vi "Photon Counter Control Panel big.vi"(8 "error in (no error)":errorcluster) -> (0 "error out":errorcluster)   [LabVIEW 2015]
uses:
  Public/Typedefs/Gate Mode.ctl
  Public/Typedefs/Discriminator Output.ctl
  <vilib>/Instr/_visa.llb/VISA GPIB Control REN Mode.ctl
  <vilib>/DAQmx/read.llb/DAQmx Read (Analog 1D DBL 1Chan NSamp).vi
  <vilib>/DAQmx/read.llb/DAQmx Read (Analog DBL 1Chan 1Samp).vi
  <vilib>/DAQmx/create/channels.llb/DAQmx Create Channel (AI-Voltage-Basic).vi
  <vilib>/Waveform/WDTFileIO.llb/Export Waveforms To Spreadsheet File (1D).vi
  <vilib>/DAQmx/miscellaneous.llb/DAQmx Fill In Error Info.vi
  SR400.lvlib
panel:
  out "PMT":dbl(graph)=0.0005292442580582076
  out "Wavemeter":dbl(graph)
  in  "file path":path=path "C:/Users/physics/Desktop/tessttt.xls"
  out "Scanning":bool
  out "Scan Finished":bool=TRUE
  out "Current Period":dbl=1.0
  out "Counter A":dbl(graph)=191.0
  out "Counter B":dbl(graph)
  in  "Monitor":bool
  in  "Start Scan":bool caption="Start Monitored Scan"
  in  "Stop Scan":bool
  out "Scan Start Time":timestamp=timestamp(3614449169.8747206 s since 1904-01-01)
  out "Counter A":dbl(graph)=5052.0
  out "Counter B":dbl(graph)=5104.0
  in  "Read Buffer Data":bool
  in  "Query Status Byte":bool
  out "Scan Start Time":timestamp=timestamp(3611333596.390047 s since 1904-01-01)
  in  "GPIB Address":i32=23 min=0 max=30 step=1
  in  "Stop Unmonitored Scan":bool
  in  "Disc A Mode":T1
  in  "Disc B Mode":T1
  in  "Disc B Slope":enum16{"Rise", "Fall"}(ring)
  in  "Disc A Slope":enum16{"Rise", "Fall"}(ring)
  in  "Trigger Slope":enum16{"Rise", "Fall"}(ring)
  in  "Set Gate Widths":bool
  in  "Set Gate Mode":bool
  out "Current":dbl[unit]=0.5 caption="Current Dwell Time"
  in  "Setpoint":dbl[unit]=0.5 caption="Dwell Time Target" min=0.0 max=60.0 step=0.5 format="%#_1g"
  in  "Set Dwell Time":bool
  in  "Setpoint":i32=5 caption="Number of Periods Target" min=0 max=2000 step=1
  out "Current":dbl=5.0 caption="Number of Periods Current"
  in  "Set # Periods":bool
  in  "Scan End Mode":enum16{"Stop", "Start"}(ring)
  in  "Disc B Lvl":dbl=-0.012 format="%#_13g"
  in  "Disc A Lvl":dbl=-0.012 format="%#_13g"
  in  "Display Mode":enum16{"Continuous", "Hold"}(ring)
  in  "Initialize":bool
  in  "Internal / External":bool
  in  "Set Count Time":bool
  in  "Counter B Input":enum16{"10 MHz", "INPUT 1", "INPUT 2", "TRIG"}(ring)=enum."INPUT 1"
  in  "Counter A Input":enum16{"10 MHz", "INPUT 1", "INPUT 2", "TRIG"}(ring)=enum."INPUT 1"
  in  "Count Mode":T2(ring)
  in  "Trigger Level":dbl=1.25 format="%#_13g"
  in  "VISA Resource Name":refnum<visa-resource-name>="GPIB0::23::INSTR"
  in  "Photon Counter SR 400":T3={"Mode"=0, "Count Time"=5.0, "Trigger Frequency"=10000000.0, "Trigger External?"=FALSE, "Gate A Mode"=0, "Gate A Width"=0.0002, "Gate A Delay"=0.0, "Gate B Mode"=0, "Gate B Width"=5e-09, "Gate B Delay"=0.0} {"Mode" items=["A,B For T Preset", "A-B For T Preset", "A+B For T Preset", "A For B Preset"]; "Gate A Mode" items=["CW", "Fixed"]; "Gate B Mode" items=["CW", "Fixed"]}
  out "Update visible/hidden":bool
  out "Current":T4
  out "Current":T4
  in  "stop":bool
  in  "Read to\nControl":bool
  in  "Read":bool
  out "Actual":dbl=200000.00000000003
  out "Actual":dbl=5.0
  in  "Target":dbl=5.0 caption="Gate A Width Percent Target"
  in  "Target":dbl=200000.00000000003 caption="Gate A Percent Target"
  in  "Gate Width: Time / Percent":bool caption="Time/Percent"
  in  "Start / Middle":bool
  in  "Setpoint":T4 caption="Gate B Mode Target"
  in  "Setpoint":T4 caption="Gate A Mode Target"
  out "Current":dbl[unit]=10000000.0 caption="Trigger Freq"
  in  "Setpoint":dbl[unit]=10000000.0 caption="Trigger Freq. Target"
  in  "Set Time & Freq.":bool
  in  "# Triggers vs Freq/Time":bool
  out "Current":dbl=50000000.0 caption="External Trigger # Cycles Current" format="%^#_6g"
  in  "Setpoint":dbl=50000000.0 format="%^#_6g"
  in  "Set # of Triggers":bool
  in  "Setpoint":dbl[unit]=5e-09 caption="Gate B Width Target"
  in  "Setpoint":dbl[unit]=0.0002 caption="Gate A Width Target"
  out "Current":dbl[unit]=0.0002 format="%^#_6g"
  out "Current":dbl[unit]=5e-09 format="%^#_6g"
  out "Current":dbl[unit]
  out "Current":dbl[unit]
  in  "Setpoint":dbl[unit]
  in  "Setpoint":dbl[unit] caption="Gate A Delay Target"
  in  "Set Gate Delays":bool
  in  "Start Unmonitored Scan":bool
  in  "Setpoint":dbl[unit]=5.0 caption="Count Time Target" min=0.0 step=0.5 format="%#_1f"
  out "Current":dbl[unit]=5.0 caption="Count Time Current" min=0.0 max=10000.0 step=1.0 format="%#_7g"
  # "SR400 Control Panel"
  # "Setup"
  # "Gates"
  # "Acquisition"
  # "Gate B Mode"
  # "# of Periods"
  # "Count Time"
  # "Gate A Mode"
  # "Gate A Width"
  # "Gate B Width"
  # "Dwell Time"
  # "Gate A Delay"
  # "Gate B Delay"
  # "Discriminator/Trigger"
  # "Set values and initialize.\n\nSettings you can \"live\" update w/o initialization:\n        All Gate Params\n        Count Time (Only largest sig digit used)\n        Dwell Time (Only largest sig digit used)\n        External Trigger\n        # Periods\n\nSettings without a \"Set _____\" button need to be changed by initialization.\n\nAll variables are initialized, but \"live\" params do not show current value until you press the set button for that parameter.\n\n\"Read\" sets the \"Current\" indicators to what the hardware has set.\n\n\"Read to Control\" sets the \"Setpoint\" controls to the values from \"Read\""
  # "Warning, saving data clears chart histories"
  # "External Trigger # of Cycles/Freq"
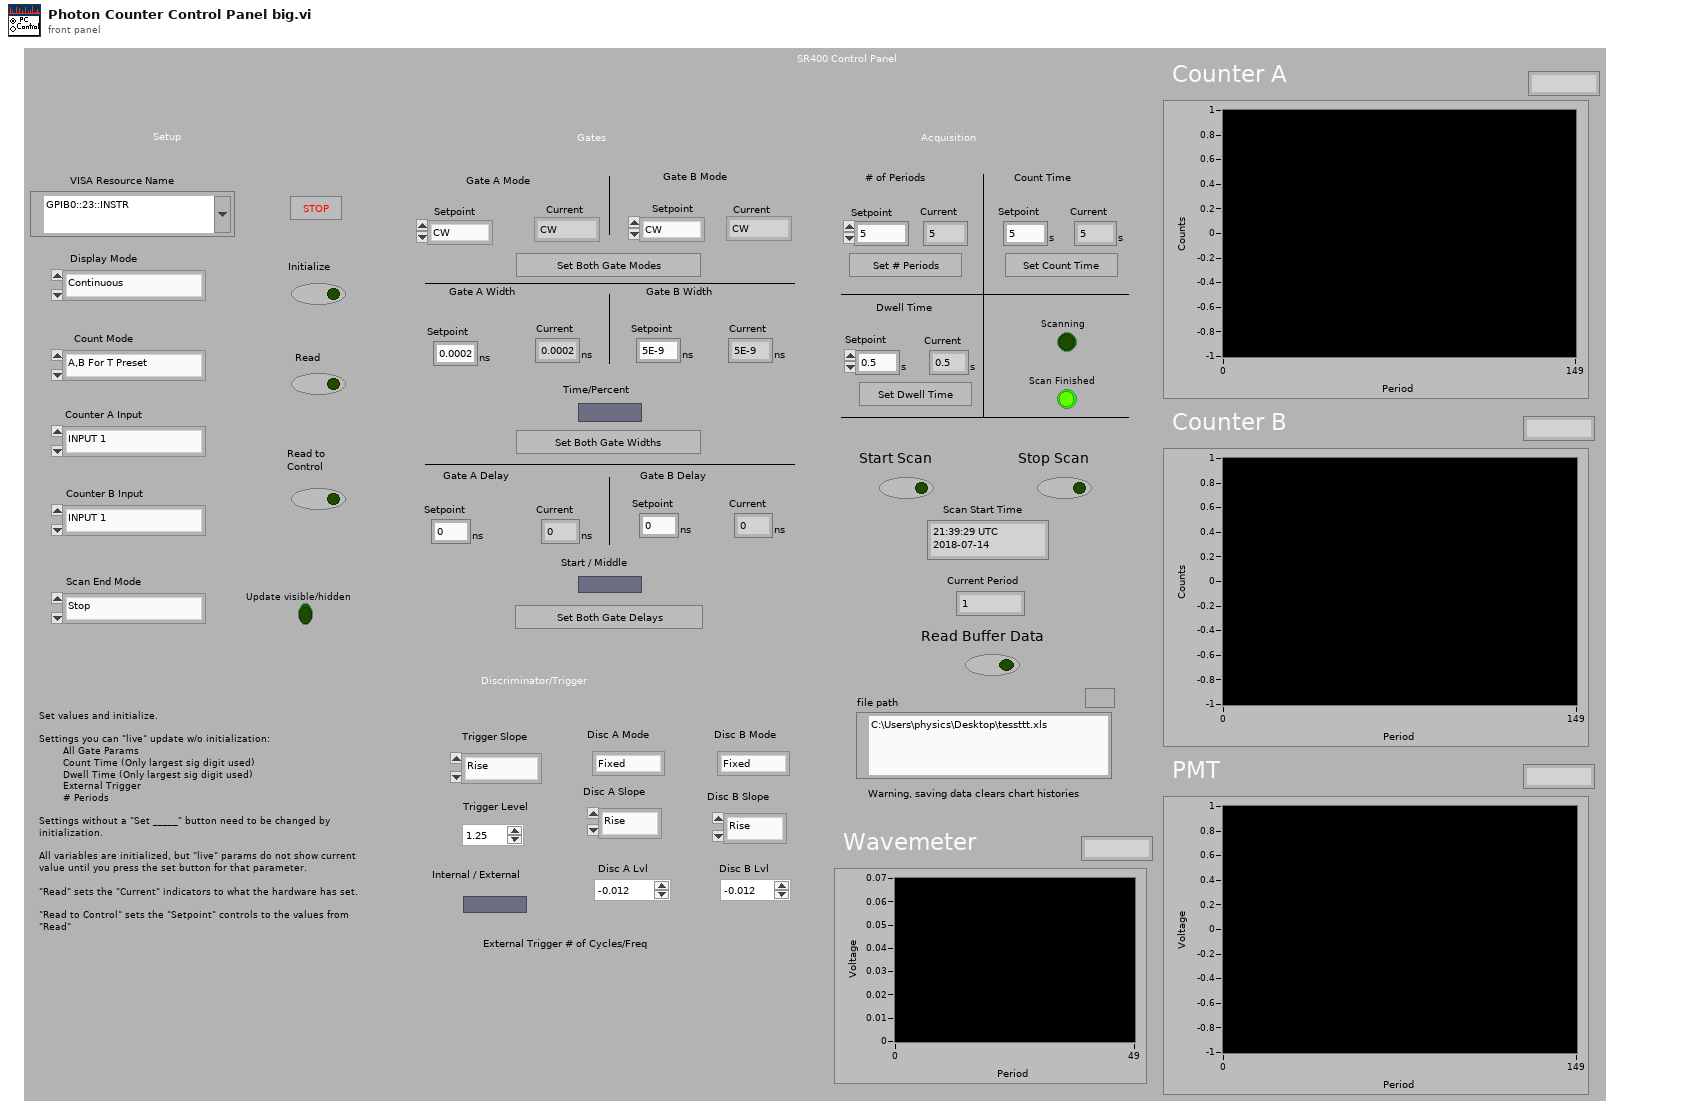
[diagram p1: front panel]
types:
  T1 = typedef "SR400.lvlib/Discriminator Output.ctl" = enum16{"Fixed", "Scan"}
  T2 = enum16{"A,B For T Preset", "A-B For T Preset", "A+B For T Preset", "A For B Preset"}
  T3 = cluster{"Mode":u16, "Count Time":dbl[unit], "Trigger Frequency":dbl[unit], "Trigger External?":bool, "Gate A Mode":u16, "Gate A Width":dbl[unit], "Gate A Delay":dbl[unit], "Gate B Mode":u16, "Gate B Width":dbl[unit], "Gate B Delay":dbl[unit]}
  T4 = typedef "SR400.lvlib/Gate Mode.ctl" = enum16{"CW", "Fixed", "Scan"}
  T5 = typedef "VISA GPIB Control REN Mode.ctl" = u16
  T6 = cluster{"Parameter Changed from front panel":bool, "Data Ready":bool, "Scan Finished":bool, "Counter Overrun":bool, "Rate Error":bool, "Recall Error":bool, "Service Request":bool, "Command Error":bool, "Triggered":bool, "Inhibited":bool, "Counting":bool}
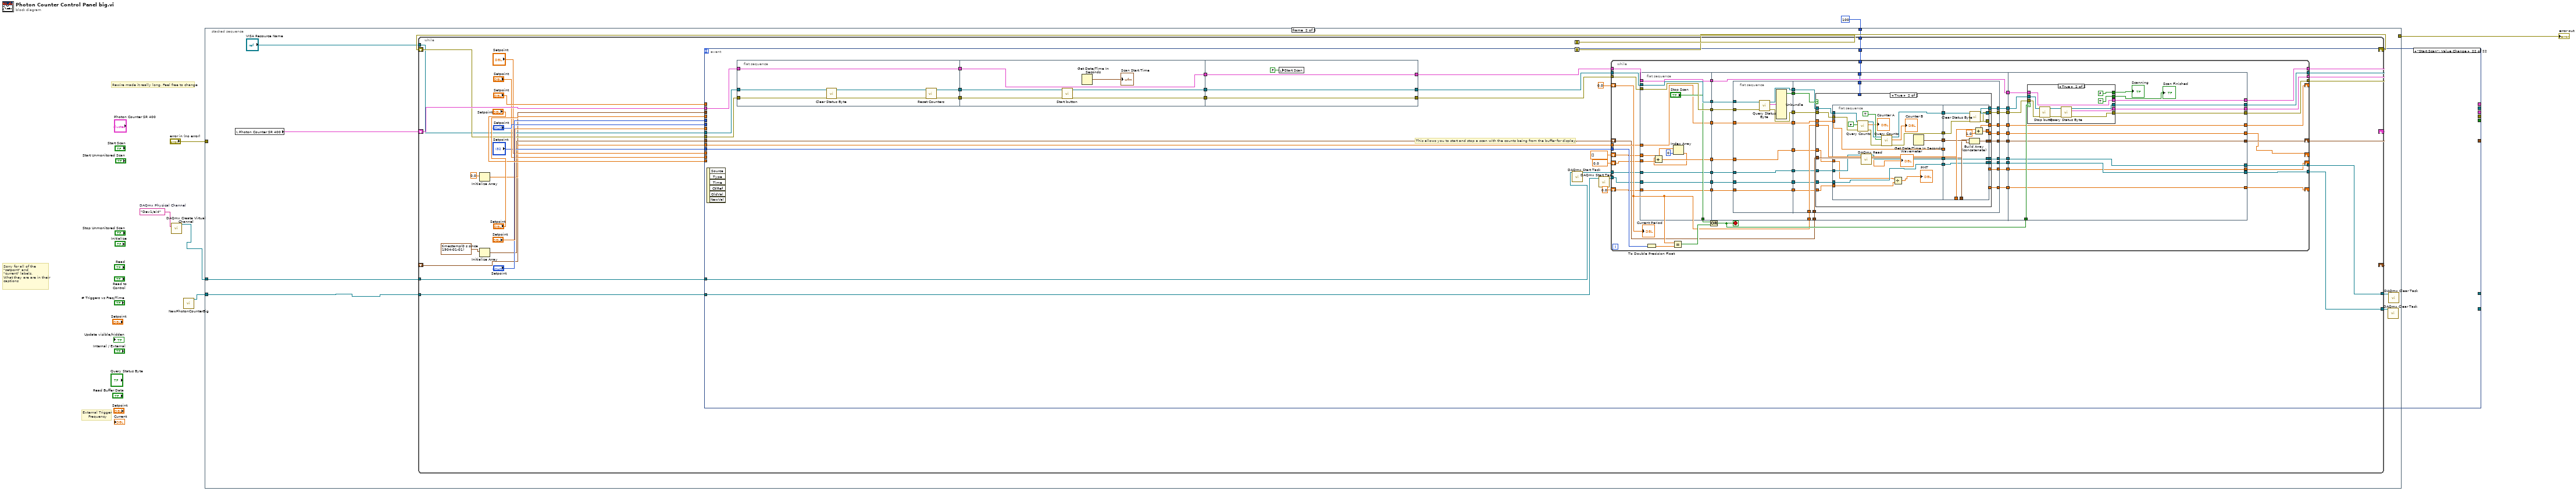
[diagram p0: block diagram]
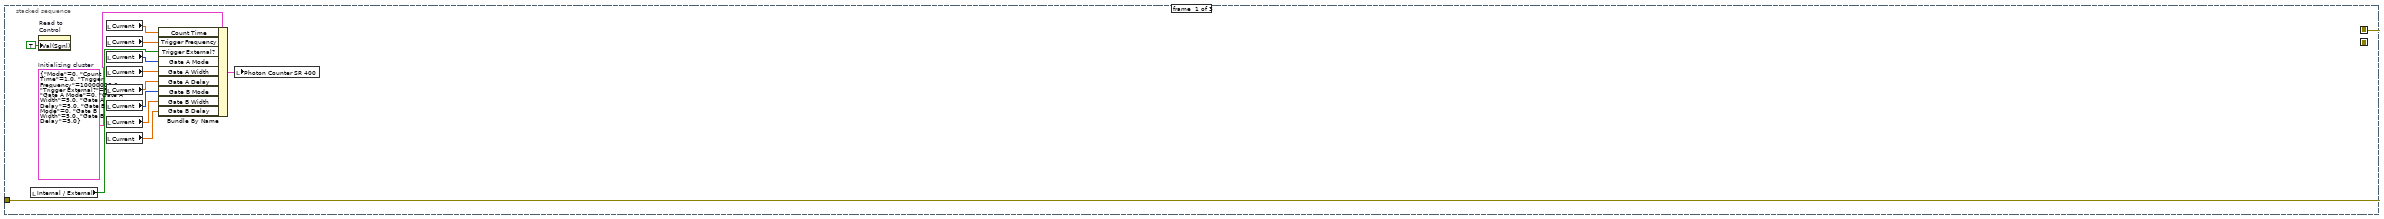
[diagram p2: hidden frame]
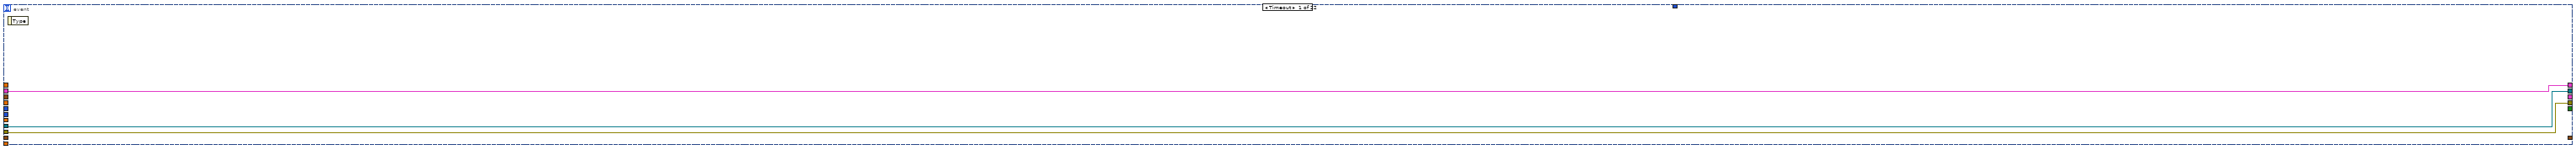
[diagram p3: hidden frame]
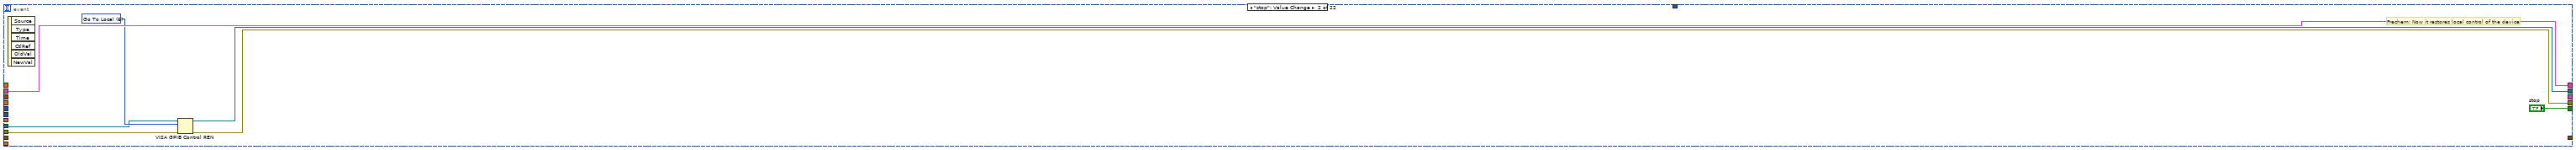
[diagram p4: hidden frame]
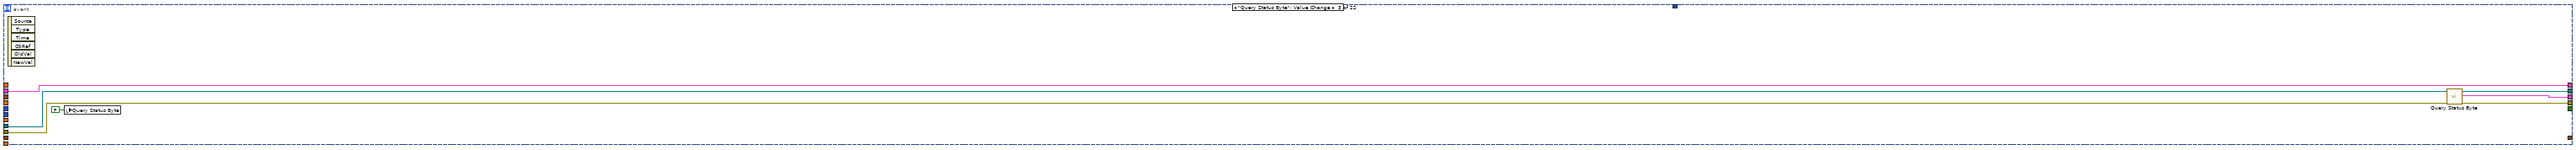
[diagram p5: hidden frame]
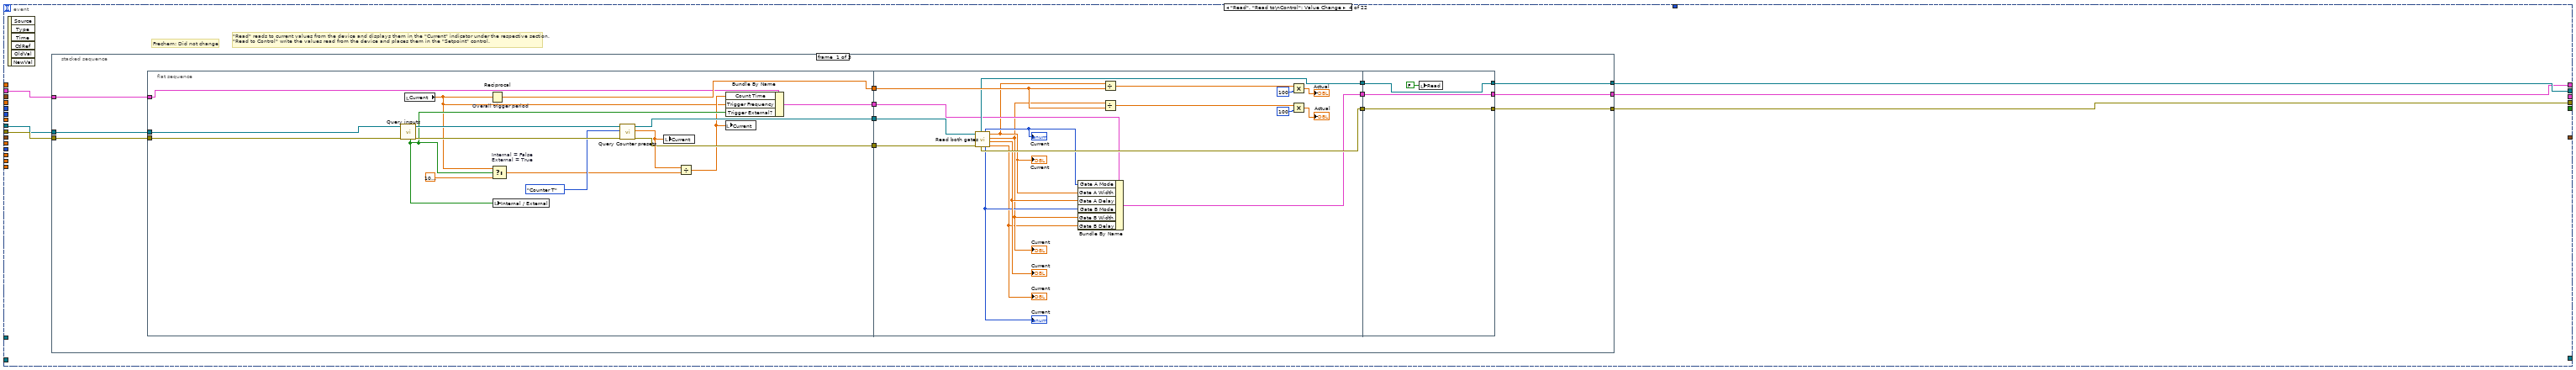
[diagram p6: hidden frame]
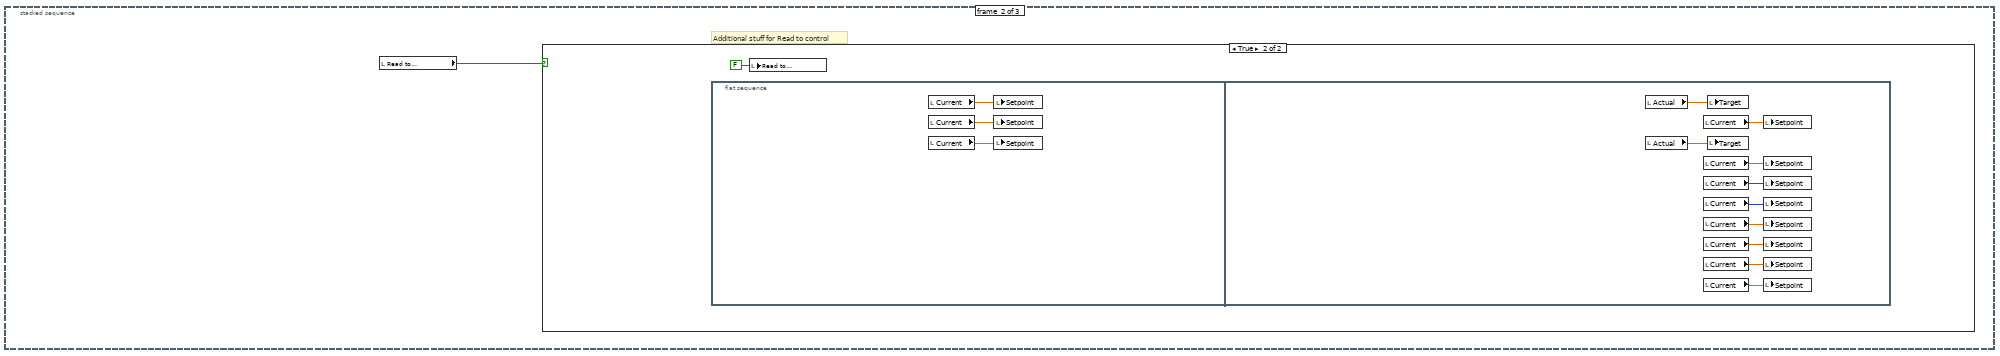
[diagram p7: hidden frame]
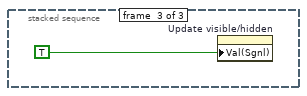
[diagram p9: hidden frame]
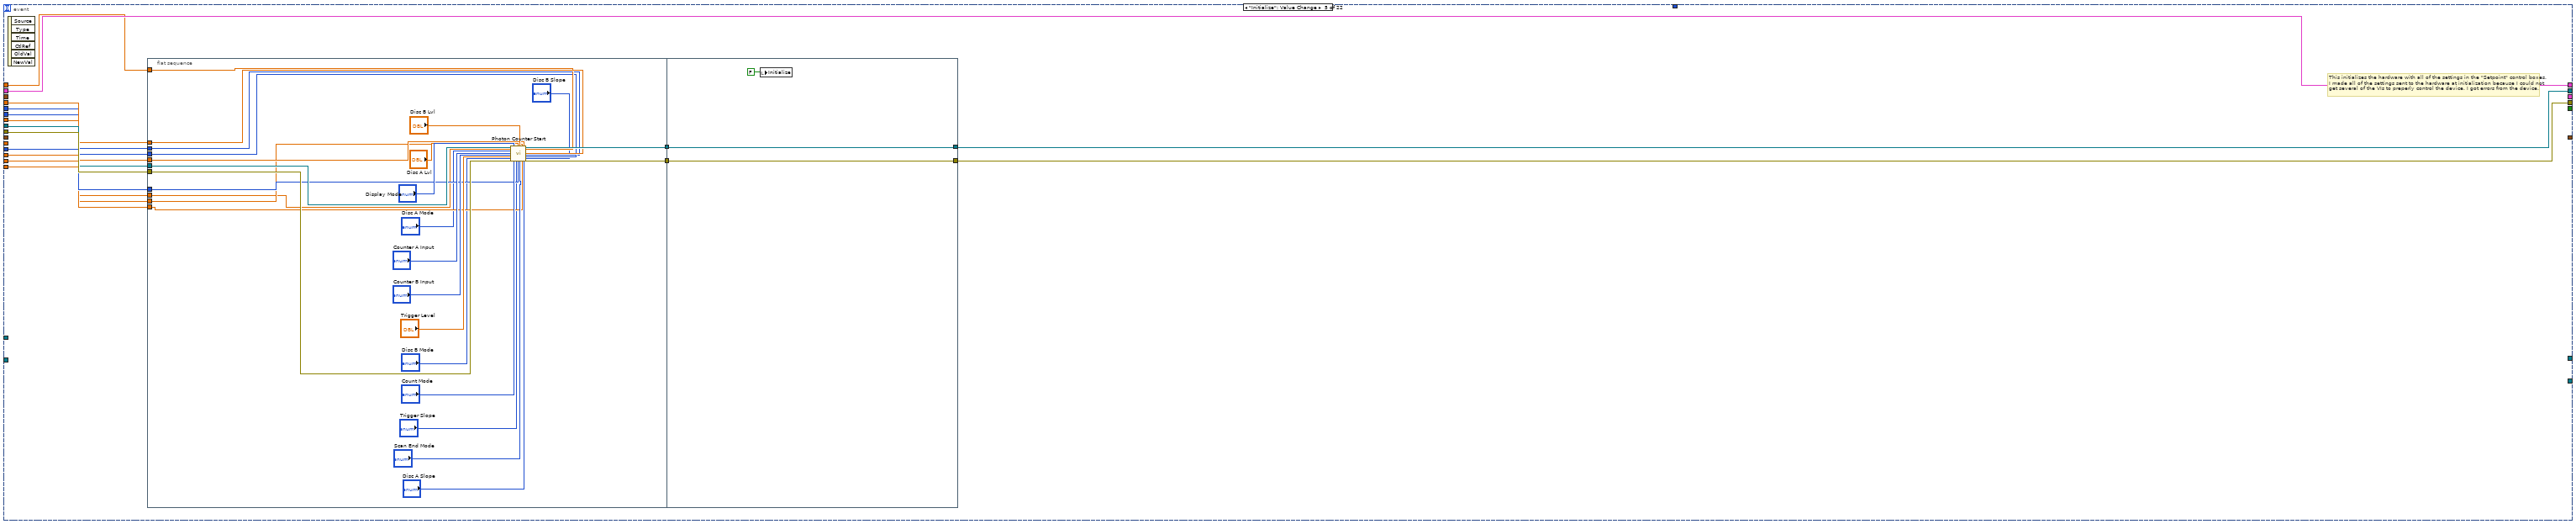
[diagram p10: hidden frame]
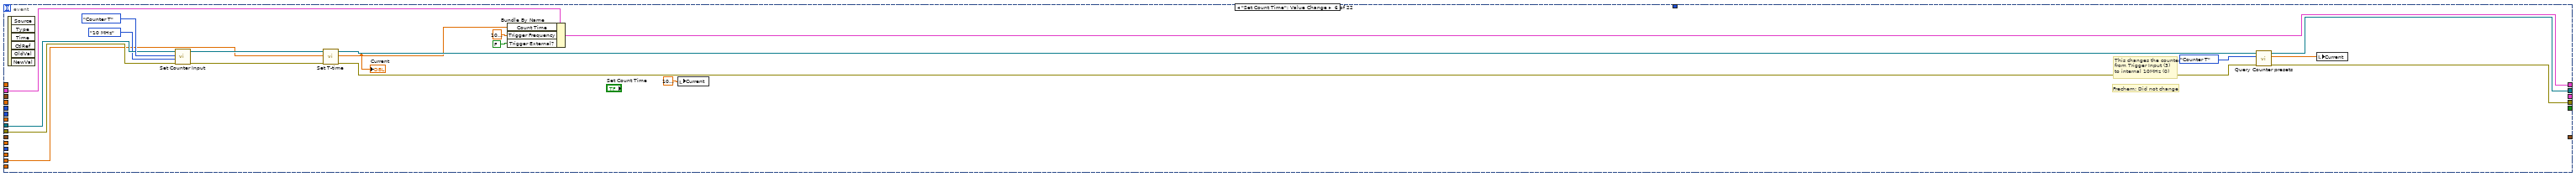
[diagram p11: hidden frame]
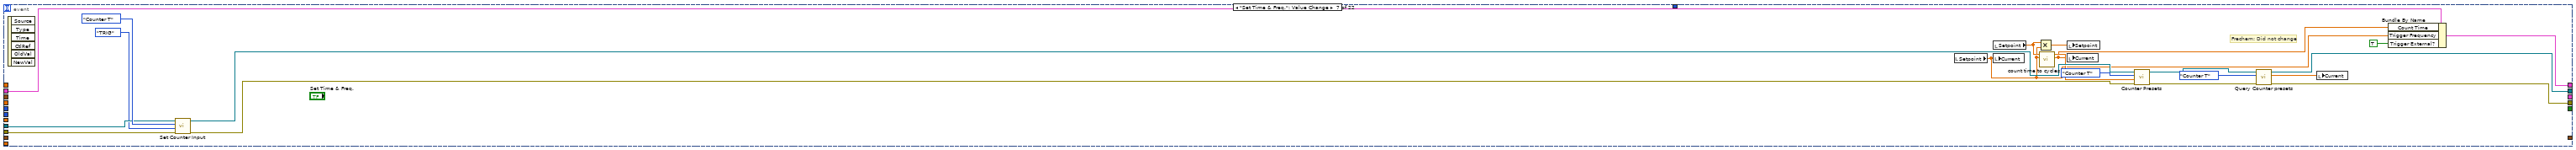
[diagram p12: hidden frame]
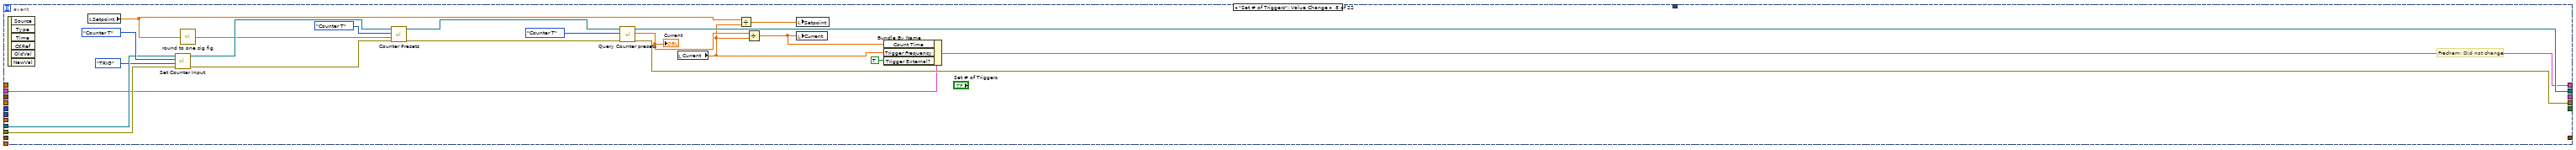
[diagram p13: hidden frame]
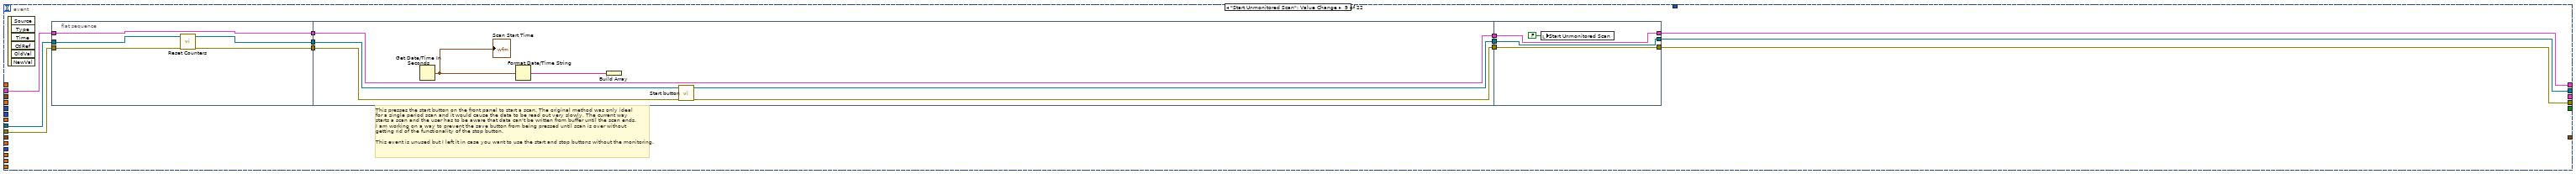
[diagram p14: hidden frame]
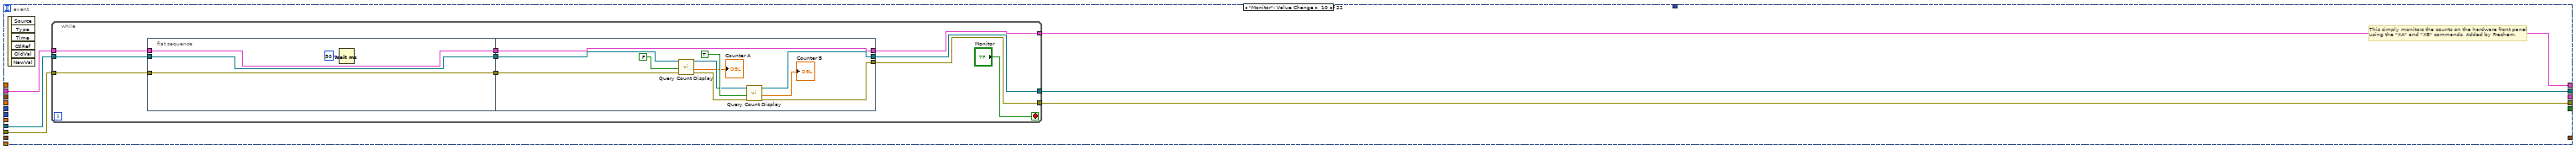
[diagram p15: hidden frame]
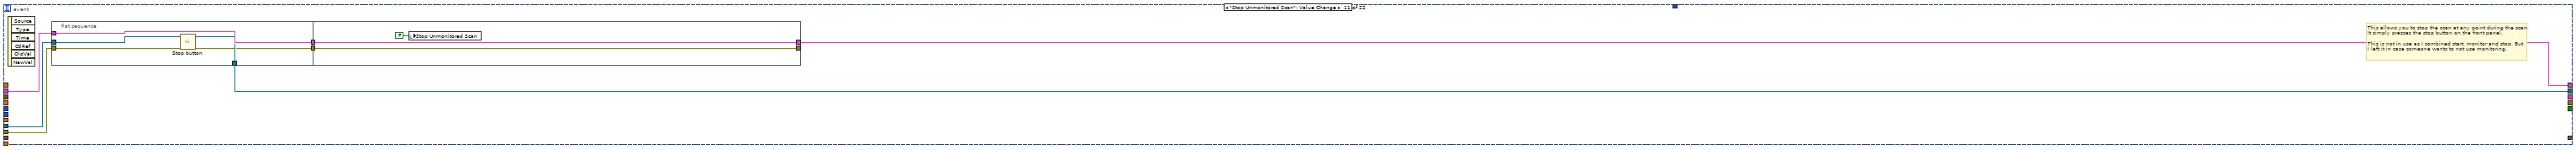
[diagram p16: hidden frame]
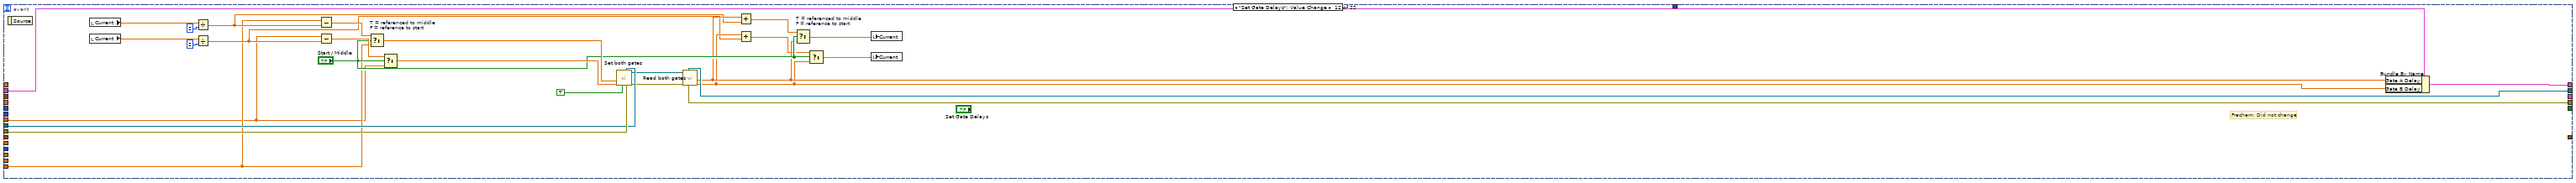
[diagram p17: hidden frame]
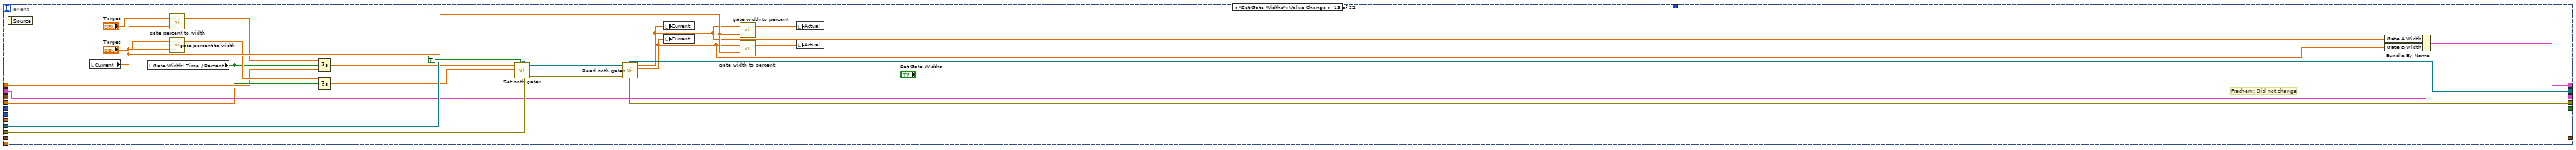
[diagram p18: hidden frame]
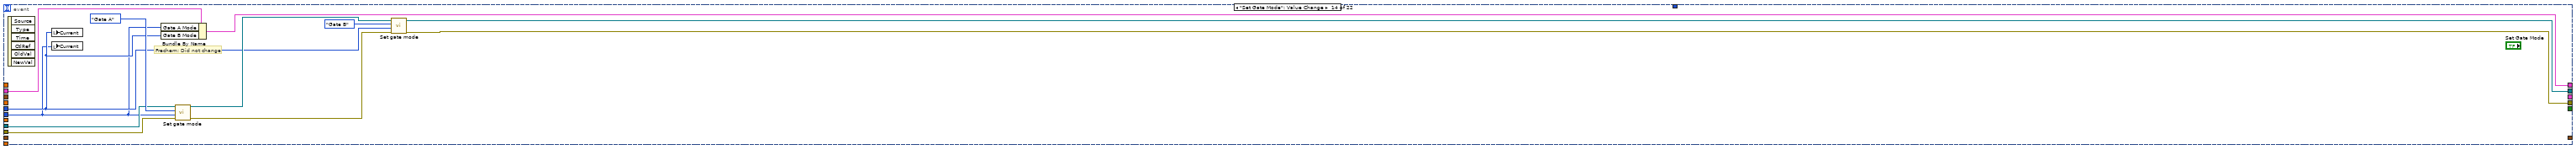
[diagram p19: hidden frame]
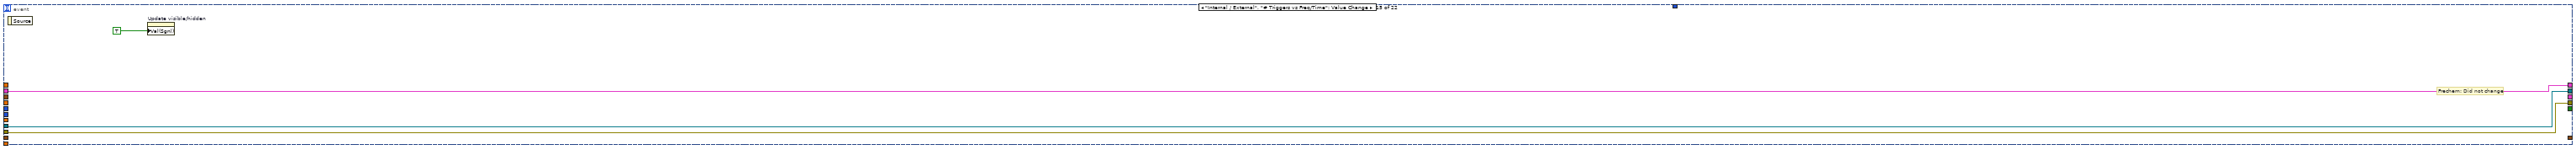
[diagram p20: hidden frame]
diagram:
  w2 = tag "Dev1/ai4"  # DAQmx Physical Channel
  # "Rewire made it really long. Feel free to change"
  # "Sorry for all of the\n\"setpont\" and \n\"current\" labels. \nWhat they are are in their\ncaptions"
  # "External Trigger \n     Frequency"
  n1 = call-poly <vilib>:"DAQmx Create Virtual Channel.vi"("physical channels"=w2) -> ("task out"=w1:refnum<k21>)  [unwired: 13 in, 1 out]
  n2 = call "NewPhotonCounterBig.vi"() -> ("task out"=w3:refnum<k21>)  [unwired: 10 in, 1 out]
  n3 = stacked-sequence {
    seq-local: [w9 _ _] -> [_ w28 _]
    seq-local: [_ w27 _] -> [_ _ w833]
    tunnel: "error in (no error)" -> [w9 _ _]
    tunnel: [_ _ w833] -> w5
    tunnel: 100 ("number of samples per channel") -> [_ w22 _]
    tunnel: w3 -> [_ w21 _]
    tunnel: w1 -> [_ w20 _]
    frame #0 {
      w7 = T3 {"Mode"=0, "Count Time"=1.0, "Trigger Frequency"=10000000.0, "Trigger External?"=FALSE, "Gate A Mode"=0, "Gate A Width"=5.0, "Gate A Delay"=5.0, "Gate B Mode"=0, "Gate B Width"=5.0, "Gate B Delay"=5.0}  # Initializing cluster
      n4 = local read "Internal / External"() -> (w16:bool)
      n5 = property on="Read to\nControl" class="Bool (strict)"("Val(Sgnl)"=TRUE ("Value (Signaling)")) -> ()  [unwired: 2 in, 2 out]
      n6 = local read "Current"() -> (w18:dbl[unit])
      n7 = local read "Current"() -> (w17:dbl[unit])
      n8 = local read "Current"() -> (w15:T4)
      n9 = local read "Current"() -> (w14:dbl[unit])
      n10 = local read "Current"() -> (w13:dbl[unit])
      n11 = local read "Current"() -> (w10:T4)
      n12 = local read "Current"() -> (w11:dbl[unit])
      n13 = local read "Current"() -> (w12:dbl[unit])
      n14 = Bundle By Name(cluster=w7, "Count Time"=w18, "Trigger Frequency"=w17, "Trigger External?"=w16, "Gate A Mode"=w15, "Gate A Width"=w14, "Gate A Delay"=w13, "Gate B Mode"=w10, "Gate B Width"=w11, "Gate B Delay"=w12) -> (w8:T3)
      n15 = local write "Photon Counter SR 400"(w8) -> ()
    }
    frame #1 {
      n16 = local read "Photon Counter SR 400"() -> (w26:T3)
      n17 = while {
        shift-right: [w52] -> _
        shift-left: w26 -> [w51]
        shift-right: [w54] -> w27
        shift-left: w28 -> [w42]
        tunnel: "VISA Resource Name" -> [w41]
        shift-right: [w35] -> _
        shift-left: _ -> [w34]
        tunnel: w20 -> [w33]
        tunnel: [w32] -> w24
        tunnel: [w31] -> w23
        tunnel: w21 -> [w30]
        tunnel: w22 -> [w29]
        stop <- w53 stop-if-true
        n18 = Initialize Array(0.0 ("element")) -> (w38:dbl[])  [unwired: 1 in]
        n19 = Initialize Array(timestamp(0 s since 1904-01-01)) -> (w36:timestamp[])  [unwired: 1 in]
        n20 = event shown="[21] \"Start Scan\": Value Change" {
          selector: _ -> [_ _ _ _ _ _ _ _ _ _ _ _ _ _ _ _ _ _ _ _ _ _]
          dyn-events: _ -> [_ _ _ _ _ _ _ _ _ _ _ _ _ _ _ _ _ _ _ _ _ _]
          timeout: _ -> [_ _ _ _ _ _ _ _ _ _ _ _ _ _ _ _ _ _ _ _ _ _]
          tunnel: [w57 w59 w67 w76 w158 w208 w226 w250 w260 w285 w313 w340 w372 w382 w393 w396 w422 w455 w471 w478 w503 w582] -> _
          tunnel: w42 -> [w56 w62 w69 w78 w162 w199 w220 w242 w264 w284 w316 w354 w373 w386 w392 w394 w421 w454 w468 w484 w506 w585]
          tunnel: [w56 w61 w68 w75 w161 w207 w227 w249 w262 w286 _ w338 w371 w383 w392 w395 w421 w454 w470 w477 w505 w584] -> w55
          tunnel: w41 -> [w57 w60 w70 w77 w156 w200 w221 w243 w256 w283 w315 w353 w374 w387 w393 w396 w422 w455 w469 w485 w504 w586]
          tunnel: w51 -> [w58 w64 w72 w74 w157 w197 w215 w236 w258 w282 w314 w352 w360 w381 w391 w397 w423 w453 w467 w476 w502 w587]
          tunnel: [w58 w64 w72 w73 w157 w196 w214 w235 w257 w281 w312 w351 w359 w380 w391 w397 w423 w453 w467 w476 w501 w583] -> w52
          tunnel: [_ "stop" _ _ _ _ _ _ _ _ _ _ _ _ _ _ _ _ _ _ _ _] -> w53
          tunnel: "Setpoint" -> [_ _ _ _ w155 _ _ _ _ _ _ _ _ _ _ _ _ _ w466 _ w500 w578]
          tunnel: "Setpoint" -> [_ _ _ _ w154 _ _ _ _ _ _ _ w356 _ _ _ _ _ _ _ _ _]
          tunnel: "Setpoint" -> [_ _ _ _ w153 _ _ _ _ _ _ _ w355 _ _ _ _ _ _ _ _ _]
          tunnel: "Setpoint" -> [_ _ _ _ w152 _ _ _ _ _ _ w328 _ _ _ _ _ _ _ _ _ _]
          tunnel: "Setpoint" -> [_ _ _ _ w151 _ _ _ _ _ _ w327 _ _ _ _ _ _ _ _ _ _]
          tunnel: "Setpoint" -> [_ _ _ _ w150 w192 _ _ _ _ _ _ _ _ _ _ _ _ _ _ w488 _]
          tunnel: "Setpoint" -> [_ _ _ _ w148 _ _ _ _ _ _ _ _ w379 _ _ _ _ _ _ _ _]
          tunnel: "Setpoint" -> [_ _ _ _ w149 _ _ _ _ _ _ _ _ w378 _ _ _ _ _ _ _ _]
          tunnel: "Setpoint" -> [_ _ _ _ w147 _ _ _ _ _ _ _ _ _ _ _ _ _ _ w482 w489 _]
          tunnel: [_ _ w66 _ _ _ _ _ _ _ _ _ _ _ _ _ _ _ _ _ _ w581] -> _
          tunnel: w38 -> [_ _ _ _ _ _ _ _ _ _ _ _ _ _ _ _ _ _ _ _ _ w579]
          tunnel: w36 -> [_ _ _ _ _ _ _ _ _ _ _ _ _ _ _ _ _ _ _ _ _ w577]
          tunnel: [_ _ _ _ _ _ _ _ _ _ _ _ _ _ _ _ _ _ _ _ _ w576] -> w35
          tunnel: w34 -> [_ _ _ _ _ _ _ _ _ _ _ _ _ _ _ _ _ _ _ _ w490 _]
          tunnel: w33 -> [_ _ _ _ _ _ _ _ _ _ _ _ _ _ _ _ _ _ _ _ _ w567]
          tunnel: [_ _ _ _ _ _ _ _ _ _ _ _ _ _ _ _ _ _ _ _ _ w575] -> w32
          tunnel: [_ _ _ _ _ _ _ _ _ _ _ _ _ _ _ _ _ _ _ _ _ w574] -> w31
          tunnel: w30 -> [_ _ _ _ _ _ _ _ _ _ _ _ _ _ _ _ _ _ _ _ _ w569]
          tunnel: w29 -> [_ _ _ _ _ _ _ _ _ _ _ _ _ _ _ _ _ _ _ _ _ w573]
          event Timeout {
            n21 = event-data() -> ()  [unwired: 2 out]
          }
          event "stop": Value Change {
            w63 = T5 6 items=["Deassert REN", "Assert REN", "Go To Local; Deassert REN ", "Assert REN; Address Device", "Local Lockout (Addressed Devices)", "Local Lockout (This Device)", "Go To Local"] ("Mode")
            # "Frechem: Now it restores local control of the device"
            n22 = event-data() -> ()  [unwired: 7 out]
            n23 = VISA GPIB Control REN(8:w62, 10:w63, 11:w60) -> (0:w61:errorcluster, 3:w59:refnum<visa-resource-name>)
          }
          event "Query Status Byte": Value Change {
            n24 = event-data() -> ()  [unwired: 7 out]
            n25 = local write "Query Status Byte"(FALSE ("Read Channels")) -> ()
            n26 = call "Query Status Byte.vi"("error in (no error)"=w69, "VISA resource name"=w70) -> ("error out"=w68:errorcluster, "Status Register"=w66:T6, "VISA resource name out"=w67:refnum<visa-resource-name>)  [unwired: 7 in]
          }
          event "Read", "Read to\nControl": Value Change {
            # "Frechem: Did not change"
            # "\"Read\" reads to current values from the device and displays them in the \"Current\" indicator under the respective section.\n\"Read to Control\" write the values read from the device and places them in the \"Setpoint\" control."
            n27 = event-data() -> ()  [unwired: 7 out]
            n28 = stacked-sequence {
              tunnel: w78 -> [w90 _ _]
              tunnel: w77 -> [w91 _ _]
              tunnel: [w86 _ _] -> w76
              tunnel: [w84 _ _] -> w75
              tunnel: w74 -> [w82 _ _]
              tunnel: [w80 _ _] -> w73
              frame #0 {
                n29 = flat-sequence {
                  tunnel: w91 -> [w107]
                  tunnel: w90 -> [w104]
                  tunnel: [w100] -> w89
                  tunnel: [w99] -> w88
                  tunnel: [w98] -> w87
                  tunnel: w82 -> [w96]
                  tunnel: [w92] -> w81
                  tunnel: w89 -> [w120]
                  tunnel: w88 -> [w119]
                  tunnel: w87 -> [w118]
                  tunnel: [w117] -> w85
                  tunnel: [w116] -> w83
                  tunnel: w81 -> [w115]
                  tunnel: [w108] -> w79
                  tunnel: [w129] -> w86
                  tunnel: w85 -> [w129]
                  tunnel: [w128] -> w84
                  tunnel: w83 -> [w128]
                  tunnel: [w127] -> w80
                  tunnel: w79 -> [w127]
                  frame #0 {
                    n30 = call "Query inputs.vi"("error in (no error)"=w104, "VISA resource name"=w107) -> ("error out"=w105:errorcluster, "VISA resource name out"=w106:refnum<visa-resource-name>, "Externally-triggered?"=w95:bool)  [unwired: 7 out]
                    n31 = local read "Current"() -> (w93:dbl[unit])
                    n32 = Reciprocal "Overall trigger period"(x=w93) -> (1/x=w98:dbl[unit])
                    n33 = Select "Internal = False\nExternal = True"(t=w93, s=w95, f=dbl[unit] 10000000.0 ("freq")) -> (s? t:f=w102:dbl[unit])
                    n34 = local write "Internal / External"(w95) -> ()
                    n35 = call "Query Counter presets.vi"("error in (no error)"=w105, "Counter (Def: T)"=enum16{"Invalid", "Counter B", "Counter T"}."Counter T" ("i (0)"), "VISA resource name"=w106) -> ("error out"=w99:errorcluster, "Number of triggers"=w101:dbl, "VISA resource name out"=w100:refnum<visa-resource-name>)  [unwired: 6 out]
                    n36 = local write "Current"(w101) -> ()
                    n37 = Divide(x=w101, y=w102) -> (x/y=w94:dbl[unit])
                    n38 = Bundle By Name(cluster=w96, "Count Time"=w94, "Trigger Frequency"=w93, "Trigger External?"=w95) -> (w92:T3)
                    n39 = local write "Current"(w94) -> ()
                  }
                  frame #1 {
                    n40 = call "Read both gates.vi"("error in (no error)"=w119, "VISA resource name"=w120) -> ("Gate B Delay"=w109:dbl[unit], "Gate A Delay"=w112:dbl[unit], "Gate B Width"=w110:dbl[unit], "Gate A Width"=w113:dbl[unit], "Current mode B"=w111:enum16{"CW", "Fixed", "Scan"}, "Current mode A"=w114:enum16{"CW", "Fixed", "Scan"}, "error out"=w116:errorcluster, "VISA resource name out"=w117:refnum<visa-resource-name>)  [unwired: 2 out]
                    "Current" <- w110
                    "Current" <- w113
                    "Current" <- w112
                    "Current" <- w109
                    "Current" <- w114
                    "Current" <- w111
                    n41 = Bundle By Name(cluster=w115, "Gate A Mode"=w114, "Gate A Width"=w113, "Gate A Delay"=w112, "Gate B Mode"=w111, "Gate B Width"=w110, "Gate B Delay"=w109) -> (w108:T3)
                    n42 = Divide(x=w113, y=w118) -> (x/y=w122:dbl)
                    n43 = Divide(x=w110, y=w118) -> (x/y=w124:dbl)
                    n44 = Multiply(x=w122, y=i8 100) -> (x*y=→"Actual":dbl)
                    n45 = Multiply(x=w124, y=i8 100) -> (x*y=→"Actual":dbl)
                  }
                  frame #2 {
                    n46 = local write "Read"(FALSE ("Read")) -> ()
                  }
                }
              }
              frame #1 {
                # "Additional stuff for Read to control"
                n47 = local read "Read to\nControl"() -> (w131:bool)
                n48 = case shown="True" w131 {
                  frame False {
                  }
                  frame True {
                    n49 = flat-sequence {
                      frame #0 {
                        n50 = local read "Current"() -> (w134:dbl)
                        n51 = local read "Current"() -> (w133:dbl[unit])
                        n52 = local read "Current"() -> (w135:dbl[unit])
                        n53 = local write "Setpoint"(w134) -> ()
                        n54 = local write "Setpoint"(w133) -> ()
                        n55 = local write "Setpoint"(w135) -> ()
                      }
                      frame #1 {
                        n56 = local read "Actual"() -> (w142:dbl)
                        n57 = local read "Actual"() -> (w144:dbl)
                        n58 = local read "Current"() -> (w137:dbl[unit])
                        n59 = local read "Current"() -> (w138:dbl[unit])
                        n60 = local read "Current"() -> (w140:T4)
                        n61 = local read "Current"() -> (w139:T4)
                        n62 = local read "Current"() -> (w143:dbl[unit])
                        n63 = local read "Current"() -> (w141:dbl[unit])
                        n64 = local read "Current"() -> (w145:dbl[unit])
                        n65 = local read "Current"() -> (w136:dbl[unit])
                        n66 = local write "Target"(w142) -> ()
                        n67 = local write "Target"(w144) -> ()
                        n68 = local write "Setpoint"(w137) -> ()
                        n69 = local write "Setpoint"(w138) -> ()
                        n70 = local write "Setpoint"(w140) -> ()
                        n71 = local write "Setpoint"(w139) -> ()
                        n72 = local write "Setpoint"(w143) -> ()
                        n73 = local write "Setpoint"(w141) -> ()
                        n74 = local write "Setpoint"(w145) -> ()
                        n75 = local write "Setpoint"(w136) -> ()
                      }
                    }
                    n76 = local write "Read to\nControl"(FALSE ("Read to Control")) -> ()
                  }
                }
              }
              frame #2 {
                n77 = property on="Update visible/hidden" class="Bool (strict)"("Val(Sgnl)"=TRUE ("Value (Signaling)")) -> ()  [unwired: 2 in, 2 out]
              }
            }
          }
          event "Initialize": Value Change {
            # "This initializes the hardware with all of the settings in the \"Setpoint\" control boxes.\nI made all of the settings sent to the hardware at initialization because I could not \nget several of the VIs to preperly control the device. I got errors from the device."
            n78 = event-data() -> ()  [unwired: 7 out]
            n79 = flat-sequence {
              tunnel: w162 -> [w188]
              tunnel: [w187] -> w160
              tunnel: [w186] -> w159
              tunnel: w156 -> [w185]
              tunnel: w155 -> [w176]
              tunnel: w154 -> [w175]
              tunnel: w153 -> [w174]
              tunnel: w152 -> [w173]
              tunnel: w151 -> [w172]
              tunnel: w150 -> [w171]
              tunnel: w149 -> [w170]
              tunnel: w148 -> [w169]
              tunnel: w147 -> [w168]
              tunnel: [w190] -> w161
              tunnel: [w191] -> w158
              tunnel: w160 -> [w191]
              tunnel: w159 -> [w190]
              frame #0 {
                n80 = call "Photon Counter Start.vi"("VISA resource name"=w185, "Dwell Time"=w168, "Disc A Mode"="Disc A Mode", "Count A Input"="Counter A Input", "Count B Input"="Counter B Input", "Trigger Level"="Trigger Level", "Disc B Mode"="Disc B Mode", "errorIN"=w188, "Display Mode"="Display Mode", "Count Mode"="Count Mode", "Trigger Slope"="Trigger Slope", "Disc A Lvl"="Disc A Lvl", "# of periods"=w176, "Disc B Lvl"="Disc B Lvl", "Scan End Mode"="Scan End Mode", "Count Time Set"=w171, "Gate A Delay (def: 0 s)"=w173, "Gate B Delay (def: 0 s)"=w172, "Disc A\nSlope"="Disc A Slope", "Gate A Width (def: 0 s)"=w174, "Gate B Width (def: 0 s)"=w175, "Gate B Mode"=w169, "Gate A Mode"=w170, "Disc B\nSlope"="Disc B Slope") -> ("VISA resource name out"=w187:refnum<visa-resource-name>, "errorOUT"=w186:errorcluster)  [unwired: 2 in]
              }
              frame #1 {
                n81 = local write "Initialize"(FALSE ("Re-initialize")) -> ()
              }
            }
          }
          event "Set Count Time": Value Change {
            # "Frechem: Did not change"
            # "This changes the counters\nfrom Trigger Input (3)\nto internal 10MHz (0)"
            n82 = event-data() -> ()  [unwired: 7 out]
            n83 = call "Set Counter Input.vi"("error in (no error)"=w199, "Input (def: 10 MHz)"=enum16{"10 MHz", "INPUT 1", "INPUT 2", "TRIG"}."10 MHz" ("n (0.000000)"), "Counter (def: A)"=enum16{"Counter A", "Counter B", "Counter T"}."Counter T" ("i (0) 2"), "VISA resource name"=w200) -> ("error out"=w202:errorcluster, "VISA resource name out"=w201:refnum<visa-resource-name>)  [unwired: 6 out]
            n84 = call "Set T-time.vi"("errorIN"=w202, "Count Time Set"=w192, "VISA resource name"=w201) -> ("errorOUT"=w203:errorcluster, "ttimeOUT"=w195:dbl[unit], "VISA resource name out"=w206:refnum<visa-resource-name>)  [unwired: 4 out]
            "Current" <- w195
            n85 = Bundle By Name(cluster=w197, "Count Time"=w195, "Trigger Frequency"=dbl[unit] 10000000.0, "Trigger External?"=FALSE) -> (w196:T3)
            n86 = local write "Current"(dbl[unit] 10000000.0 ("freq")) -> ()
            n87 = call "Query Counter presets.vi"("error in (no error)"=w203, "Counter (Def: T)"=enum16{"Invalid", "Counter B", "Counter T"}."Counter T" ("i (0)"), "VISA resource name"=w206) -> ("error out"=w207:errorcluster, "Number of triggers"=w209:dbl, "VISA resource name out"=w208:refnum<visa-resource-name>)  [unwired: 6 out]
            n88 = local write "Current"(w209) -> ()
          }
          event "Set Time & Freq.": Value Change {
            # "Frechem: Did not change"
            n89 = event-data() -> ()  [unwired: 7 out]
            n90 = call "Set Counter Input.vi"("error in (no error)"=w220, "Input (def: 10 MHz)"=enum16{"10 MHz", "INPUT 1", "INPUT 2", "TRIG"}."TRIG" ("n (0.000000)"), "Counter (def: A)"=enum16{"Counter A", "Counter B", "Counter T"}."Counter T" ("i (0) 2"), "VISA resource name"=w221) -> ("error out"=w222:errorcluster, "VISA resource name out"=w223:refnum<visa-resource-name>)  [unwired: 6 out]
            n91 = local read "Setpoint"() -> (w211:dbl[unit])
            n92 = local read "Setpoint"() -> (w216:dbl[unit])
            n93 = local write "Current"(w211) -> ()
            n94 = Multiply(x=w216, y=w211) -> (x*y=w217:dbl)
            n95 = call "count time to cycles.vi"("Trigger Freq"=w211, "Count Time Set"=w216) -> ("Count Time Current"=w212:dbl[unit], "Number of triggers"=w218:dbl)  [unwired: 3 in, 1 out]
            n96 = local write "Setpoint"(w217) -> ()
            n97 = local write "Current"(w212) -> ()
            n98 = call "Counter Presets.vi"("error in (no error)"=w222, "Number of triggers"=w218, "Counter (Def: T)"=enum16{"Invalid", "Counter B", "Counter T"}."Counter T" ("i (0) 2"), "VISA resource name"=w223) -> ("error out"=w228:errorcluster, "VISA resource name out"=w225:refnum<visa-resource-name>)  [unwired: 6 out]
            n99 = call "Query Counter presets.vi"("error in (no error)"=w228, "Counter (Def: T)"=enum16{"Invalid", "Counter B", "Counter T"}."Counter T" ("i (0)"), "VISA resource name"=w225) -> ("error out"=w227:errorcluster, "Number of triggers"=w229:dbl, "VISA resource name out"=w226:refnum<visa-resource-name>)  [unwired: 6 out]
            n100 = local write "Current"(w229) -> ()
            n101 = Bundle By Name(cluster=w215, "Count Time"=w212, "Trigger Frequency"=w211, "Trigger External?"=TRUE) -> (w214:T3)
          }
          event "Set # of Triggers": Value Change {
            # "Frechem: Did not change"
            n102 = event-data() -> ()  [unwired: 7 out]
            n103 = local read "Setpoint"() -> (w240:dbl)
            n104 = call "Set Counter Input.vi"("error in (no error)"=w242, "Input (def: 10 MHz)"=enum16{"10 MHz", "INPUT 1", "INPUT 2", "TRIG"}."TRIG" ("n (0.000000)"), "Counter (def: A)"=enum16{"Counter A", "Counter B", "Counter T"}."Counter T" ("i (0) 2"), "VISA resource name"=w243) -> ("error out"=w244:errorcluster, "VISA resource name out"=w245:refnum<visa-resource-name>)  [unwired: 6 out]
            n105 = call "round to one sig fig.vi"("input number"=w240) -> ("rounded to 1 sig fig"=w238:dbl)
            n106 = call "Counter Presets.vi"("error in (no error)"=w244, "Number of triggers"=w238, "Counter (Def: T)"=enum16{"Invalid", "Counter B", "Counter T"}."Counter T" ("i (0) 2"), "VISA resource name"=w245) -> ("error out"=w248:errorcluster, "VISA resource name out"=w247:refnum<visa-resource-name>)  [unwired: 6 out]
            n107 = call "Query Counter presets.vi"("error in (no error)"=w248, "Counter (Def: T)"=enum16{"Invalid", "Counter B", "Counter T"}."Counter T" ("i (0)"), "VISA resource name"=w247) -> ("error out"=w249:errorcluster, "Number of triggers"=w237:dbl, "VISA resource name out"=w250:refnum<visa-resource-name>)  [unwired: 6 out]
            "Current" <- w237
            n108 = local read "Current"() -> (w232:dbl[unit])
            n109 = Divide(x=w240, y=w232) -> (x/y=w239:dbl[unit])
            n110 = Divide(x=w237, y=w232) -> (x/y=w234:dbl[unit])
            n111 = local write "Setpoint"(w239) -> ()
            n112 = local write "Current"(w234) -> ()
            n113 = Bundle By Name(cluster=w236, "Count Time"=w234, "Trigger Frequency"=w232, "Trigger External?"=TRUE) -> (w235:T3)
          }
          event "Start Unmonitored Scan": Value Change {
            # "This presses the start button on the front panel to start a scan. The original method was only ideal\nfor a single period scan and it would cause the data to be read out very slowly. The current way \nstarts a scan and the user has to be aware that data can't be written from buffer until the scan ends.\nI am working on a way to prevent the save button from being pressed until scan is over without \ngetting rid of the functionality of the stop button.\n\nThis event is unused but I left it in case you want to use the start and stop buttons without the monitoring."
            n114 = event-data() -> ()  [unwired: 7 out]
            n115 = flat-sequence {
              tunnel: w258 -> [w269]
              tunnel: w256 -> [w268]
              tunnel: w264 -> [w266]
              tunnel: [w265] -> w255
              tunnel: [w267] -> w254
              tunnel: [w269] -> w253
              tunnel: [w275] -> w263
              tunnel: [w273] -> w261
              tunnel: [w272] -> w259
              tunnel: w255 -> [w276]
              tunnel: w254 -> [w274]
              tunnel: w253 -> [w272]
              tunnel: [w277] -> w262
              tunnel: w263 -> [w277]
              tunnel: w261 -> [w278]
              tunnel: [w278] -> w260
              tunnel: [w279] -> w257
              tunnel: w259 -> [w279]
              frame #0 {
                n116 = call "Reset Counters.vi"("error in (no error)"=w266, "VISA resource name"=w268) -> ("error out"=w265:errorcluster, "VISA resource name out"=w267:refnum<visa-resource-name>)  [unwired: 8 in]
              }
              frame #1 {
                n117 = Get Date/Time In Seconds() -> (seconds since 1Jan1904=w271:timestamp)
                "Scan Start Time" <- w271
                n118 = Format Date/Time String(seconds (now)=w271) -> (date/time string=w270:string)  [unwired: 2 in]
                n119 = Build Array(w270) -> ()  [unwired: 1 out]
                n120 = call "Start button.vi"("error in (no error)"=w276, "VISA resource name"=w274) -> ("error out"=w275:errorcluster, "VISA resource name out"=w273:refnum<visa-resource-name>)  [unwired: 8 in]
              }
              frame #2 {
                n121 = local write "Start Unmonitored Scan"(FALSE ("Read Channels")) -> ()
              }
            }
          }
          event "Monitor": Value Change {
            # "This simply monitors the counts on the hardware front panel\nusing the \"XA\" and \"XB\" commands. Added by Frechem."
            n122 = event-data() -> ()  [unwired: 7 out]
            n123 = while {
              tunnel: w282 -> [w289]
              tunnel: [w288] -> w281
              tunnel: w283 -> [w290]
              tunnel: [w292] -> w285
              tunnel: w284 -> [w291]
              tunnel: [w293] -> w286
              stop <- "Monitor" stop-if-true
              n124 = flat-sequence {
                tunnel: w290 -> [w299]
                tunnel: [w299] -> w296
                tunnel: w291 -> [w298]
                tunnel: [w298] -> w295
                tunnel: w289 -> [w297]
                tunnel: [w297] -> w294
                tunnel: w296 -> [w303]
                tunnel: w295 -> [w302]
                tunnel: w294 -> [w301]
                tunnel: [w305] -> w292
                tunnel: [w304] -> w293
                tunnel: [w301] -> w288
                frame #0 {
                  n125 = Wait (ms)(milliseconds to wait=u32 50) -> ()  [unwired: 1 out]
                }
                frame #1 {
                  n126 = call "Query Count Display.vi"("error in (no error)"=w302, "Read B?"=FALSE, "VISA resource name"=w303) -> ("error out"=w310:errorcluster, "Counts"=→"Counter A":dbl, "VISA resource name out"=w308:refnum<visa-resource-name>)  [unwired: 6 in]
                  n127 = call "Query Count Display.vi"("error in (no error)"=w310, "Read B?"=TRUE, "VISA resource name"=w308) -> ("error out"=w304:errorcluster, "Counts"=→"Counter B":dbl, "VISA resource name out"=w305:refnum<visa-resource-name>)  [unwired: 6 in]
                }
              }
            }
          }
          event "Stop Unmonitored Scan": Value Change {
            # "This allows you to stop the scan at any point during the scan. \nIt simply presses the stop button on the front panel.\n\nThis is not in use as I combined start, monitor and stop. But, \nI left it in case someone wants to not use monitoring."
            n128 = event-data() -> ()  [unwired: 7 out]
            n129 = flat-sequence {
              tunnel: w316 -> [w322]
              tunnel: w314 -> [w321]
              tunnel: [w319] -> w318
              tunnel: [w321] -> w317
              tunnel: w315 -> [w323]
              tunnel: [w320] -> w313
              tunnel: [w325] -> w312
              tunnel: [w326] -> _
              tunnel: w318 -> [w326]
              tunnel: w317 -> [w325]
              frame #0 {
                n130 = call "Stop button.vi"("error in (no error)"=w322, "VISA resource name"=w323) -> ("error out"=w319:errorcluster, "VISA resource name out"=w320:refnum<visa-resource-name>)  [unwired: 8 in]
              }
              frame #1 {
                n131 = local write "Stop Unmonitored Scan"(FALSE ("Read Channels")) -> ()
              }
            }
          }
          event "Set Gate Delays": Value Change {
            # "Frechem: Did not change"
            n132 = event-data() -> ()  [unwired: 2 out]
            n133 = local read "Current"() -> (w349:dbl[unit])
            n134 = local read "Current"() -> (w348:dbl[unit])
            n135 = Divide(x=w349, y=2) -> (x/y=w329:dbl[unit])
            n136 = Divide(x=w348, y=2) -> (x/y=w330:dbl[unit])
            n137 = Subtract(x=w328, y=w329) -> (x-y=w345:dbl[unit])
            n138 = Subtract(x=w327, y=w330) -> (x-y=w343:dbl[unit])
            n139 = Select "T = referenced to middle\nF = reference to start"(t=w345, s="Start / Middle", f=w328) -> (s? t:f=w342:dbl[unit])
            n140 = Select(t=w343, s="Start / Middle", f=w327) -> (s? t:f=w344:dbl[unit])
            n141 = call "Set both gates.vi"("Error In"=w354, "VISA resource name"=w353, "Set Delay?"=TRUE, "gatedelayoffsetB"=w344, "gatedelayoffsetA"=w342) -> ("Error Out"=w339:errorcluster, "VISA resource name out"=w341:refnum<visa-resource-name>)  [unwired: 3 in, 2 out]
            n142 = call "Read both gates.vi"("error in (no error)"=w339, "VISA resource name"=w341) -> ("Gate B Delay"=w335:dbl[unit], "Gate A Delay"=w336:dbl[unit], "error out"=w338:errorcluster, "VISA resource name out"=w340:refnum<visa-resource-name>)  [unwired: 6 out]
            n143 = Add(x=w336, y=w329) -> (x+y=w334:dbl[unit])
            n144 = Add(x=w335, y=w330) -> (x+y=w333:dbl[unit])
            n145 = Select "T = referenced to middle\nF = reference to start"(t=w334, s="Start / Middle", f=w336) -> (s? t:f=w332:dbl[unit])
            n146 = Select(t=w333, s="Start / Middle", f=w335) -> (s? t:f=w331:dbl[unit])
            n147 = local write "Current"(w332) -> ()
            n148 = local write "Current"(w331) -> ()
            n149 = Bundle By Name(cluster=w352, "Gate A Delay"=w336, "Gate B Delay"=w335) -> (w351:T3)
          }
          event "Set Gate Widths": Value Change {
            # "Frechem: Did not change"
            n150 = event-data() -> ()  [unwired: 2 out]
            n151 = local read "Current"() -> (w368:dbl[unit])
            n152 = local read "Gate Width: Time / Percent"() -> (w362:bool)
            n153 = call "gate percent to width.vi"("Trigger Freq"=w368, "Gate %"="Target") -> ("Gate width"=w364:dbl[unit])  [unwired: 1 out]
            n154 = call "gate percent to width.vi"("Trigger Freq"=w368, "Gate %"="Target") -> ("Gate width"=w363:dbl[unit])  [unwired: 1 out]
            n155 = Select(t=w364, s=w362, f=w355) -> (s? t:f=w365:dbl[unit])
            n156 = Select(t=w363, s=w362, f=w356) -> (s? t:f=w361:dbl[unit])
            n157 = call "Set both gates.vi"("Error In"=w373, "VISA resource name"=w374, "Set Width?"=TRUE, "Gate B Width"=w361, "Gate A Width"=w365) -> ("Error Out"=w377:errorcluster, "VISA resource name out"=w376:refnum<visa-resource-name>)  [unwired: 3 in, 2 out]
            n158 = call "Read both gates.vi"("error in (no error)"=w377, "VISA resource name"=w376) -> ("Gate B Width"=w357:dbl[unit], "Gate A Width"=w358:dbl[unit], "error out"=w371:errorcluster, "VISA resource name out"=w372:refnum<visa-resource-name>)  [unwired: 6 out]
            n159 = local write "Current"(w358) -> ()
            n160 = local write "Current"(w357) -> ()
            n161 = call "gate width to percent.vi"("Trigger Freq"=w368, "Gate width"=w358) -> ("Gate %"=w369:dbl)  [unwired: 1 out]
            n162 = call "gate width to percent.vi"("Trigger Freq"=w368, "Gate width"=w357) -> ("Gate %"=w370:dbl)  [unwired: 1 out]
            n163 = local write "Actual"(w369) -> ()
            n164 = local write "Actual"(w370) -> ()
            n165 = Bundle By Name(cluster=w360, "Gate A Width"=w358, "Gate B Width"=w357) -> (w359:T3)
          }
          event "Set Gate Mode": Value Change {
            # "Frechem: Did not change"
            n166 = event-data() -> ()  [unwired: 7 out]
            n167 = local write "Current"(w379) -> ()
            n168 = local write "Current"(w378) -> ()
            n169 = Bundle By Name(cluster=w381, "Gate A Mode"=w378, "Gate B Mode"=w379) -> (w380:T3)
            n170 = call "Set gate mode.vi"("error in (no error)"=w386, "Mode (def: CW)"=w378, "Gate (def: A)"=enum16{"Gate A", "Gate B"}."Gate A" ("i (0)"), "VISA resource name"=w387) -> ("error out"=w385:errorcluster, "VISA resource name out"=w384:refnum<visa-resource-name>)  [unwired: 6 out]
            n171 = call "Set gate mode.vi"("error in (no error)"=w385, "Mode (def: CW)"=w379, "Gate (def: A)"=enum16{"Gate A", "Gate B"}."Gate B" ("i (0)"), "VISA resource name"=w384) -> ("error out"=w383:errorcluster, "VISA resource name out"=w382:refnum<visa-resource-name>)  [unwired: 6 out]
          }
          event "Internal / External", "# Triggers vs Freq/Time": Value Change {
            # "Frechem: Did not change"
            n172 = event-data() -> ()  [unwired: 2 out]
            n173 = property on="Update visible/hidden" class="Bool (strict)"("Val(Sgnl)"=TRUE ("Value (Signaling)")) -> ()  [unwired: 2 in, 2 out]
          }
          event "Gate Width: Time / Percent": Value Change {
            # "Frechem: Did not change"
            # "Changes the gate widths to percents and updates values.\n\"Current\" is the value last read from the device."
            n174 = event-data() -> ("NewVal"=w398:bool)  [unwired: 6 out]
            n175 = local read "Current"() -> (w399:dbl[unit])
            n176 = property on="Update visible/hidden" class="Bool (strict)"("Val(Sgnl)"=TRUE ("Value (Signaling)")) -> ()  [unwired: 2 in, 2 out]
            n177 = case shown="True" w398 {
              tunnel: w399 -> [w404 w420]
              tunnel: [w401 w411] -> w395
              tunnel: w394 -> [w401 w411]
              frame False {
                n178 = local read "Actual"() -> (w407:dbl)
                n179 = local read "Actual"() -> (w408:dbl)
                n180 = local read "Target"() -> (w402:dbl)
                n181 = local read "Target"() -> (w403:dbl)
                n182 = call "gate percent to width.vi"("Trigger Freq"=w404, "Gate %"=w407) -> ("Gate width"=w405:dbl[unit])  [unwired: 1 out]
                n183 = call "gate percent to width.vi"("Trigger Freq"=w404, "Gate %"=w408) -> ("Gate width"=w406:dbl[unit])  [unwired: 1 out]
                n184 = call "gate percent to width.vi"("Trigger Freq"=w404, "Gate %"=w402) -> ("Gate width"=w410:dbl[unit])  [unwired: 1 out]
                n185 = call "gate percent to width.vi"("Trigger Freq"=w404, "Gate %"=w403) -> ("Gate width"=w409:dbl[unit])  [unwired: 1 out]
                n186 = local write "Current"(w405) -> ()
                n187 = local write "Current"(w406) -> ()
                n188 = local write "Setpoint"(w410) -> ()
                n189 = local write "Setpoint"(w409) -> ()
              }
              frame True {
                n190 = local read "Setpoint"() -> (w419:dbl[unit])
                n191 = local read "Setpoint"() -> (w417:dbl[unit])
                n192 = local read "Current"() -> (w415:dbl[unit])
                n193 = local read "Current"() -> (w413:dbl[unit])
                n194 = call "gate width to percent.vi"("Trigger Freq"=w420, "Gate width"=w419) -> ("Gate %"=w418:dbl)  [unwired: 1 out]
                n195 = call "gate width to percent.vi"("Trigger Freq"=w420, "Gate width"=w417) -> ("Gate %"=w416:dbl)  [unwired: 1 out]
                n196 = call "gate width to percent.vi"("Trigger Freq"=w420, "Gate width"=w415) -> ("Gate %"=w414:dbl)  [unwired: 1 out]
                n197 = call "gate width to percent.vi"("Trigger Freq"=w420, "Gate width"=w413) -> ("Gate %"=w412:dbl)  [unwired: 1 out]
                n198 = local write "Target"(w418) -> ()
                n199 = local write "Target"(w416) -> ()
                n200 = local write "Actual"(w414) -> ()
                n201 = local write "Actual"(w412) -> ()
              }
            }
          }
          event "Start / Middle": Value Change {
            # "Frechem: Did not change"
            # "Updates the gate widths depending on when it is set."
            n202 = event-data() -> ("NewVal"=w424:bool)  [unwired: 6 out]
            n203 = case shown="False" w424 {
              frame False {
                n204 = local read "Current"() -> (w438:dbl[unit])
                n205 = local read "Current"() -> (w435:dbl[unit])
                n206 = local read "Setpoint"() -> (w433:dbl[unit])
                n207 = local read "Setpoint"() -> (w428:dbl[unit])
                n208 = local read "Current"() -> (w431:dbl[unit])
                n209 = local read "Current"() -> (w426:dbl[unit])
                n210 = Divide(x=w438, y=2) -> (x/y=w434:dbl[unit])
                n211 = Divide(x=w435, y=2) -> (x/y=w429:dbl[unit])
                n212 = Subtract(x=w431, y=w434) -> (x-y=w430:dbl[unit])
                n213 = Subtract(x=w433, y=w434) -> (x-y=w432:dbl[unit])
                n214 = Subtract(x=w426, y=w429) -> (x-y=w425:dbl[unit])
                n215 = Subtract(x=w428, y=w429) -> (x-y=w427:dbl[unit])
                n216 = local write "Current"(w430) -> ()
                n217 = local write "Setpoint"(w432) -> ()
                n218 = local write "Current"(w425) -> ()
                n219 = local write "Setpoint"(w427) -> ()
              }
              frame True {
                n220 = local read "Current"() -> (w449:dbl[unit])
                n221 = local read "Current"() -> (w452:dbl[unit])
                n222 = local read "Setpoint"() -> (w442:dbl[unit])
                n223 = local read "Setpoint"() -> (w447:dbl[unit])
                n224 = local read "Current"() -> (w440:dbl[unit])
                n225 = local read "Current"() -> (w445:dbl[unit])
                n226 = Divide(x=w449, y=2) -> (x/y=w443:dbl[unit])
                n227 = Divide(x=w452, y=2) -> (x/y=w448:dbl[unit])
                n228 = Add(x=w440, y=w443) -> (x+y=w439:dbl[unit])
                n229 = Add(x=w442, y=w443) -> (x+y=w441:dbl[unit])
                n230 = Add(x=w445, y=w448) -> (x+y=w444:dbl[unit])
                n231 = Add(x=w447, y=w448) -> (x+y=w446:dbl[unit])
                n232 = local write "Current"(w439) -> ()
                n233 = local write "Setpoint"(w441) -> ()
                n234 = local write "Current"(w444) -> ()
                n235 = local write "Setpoint"(w446) -> ()
              }
            }
          }
          event "Update visible/hidden": Value Change {
            n236 = event-data() -> ()  [unwired: 7 out]
            n237 = flat-sequence {
              frame #0 {
                n238 = property on="Target" class="DigNum (strict)"("Visible"="Gate Width: Time / Percent") -> ()  [unwired: 2 in, 2 out]
                n239 = property on="Actual" class="DigNum (strict)"("Visible"="Gate Width: Time / Percent") -> ()  [unwired: 2 in, 2 out]
                n240 = property on="Actual" class="DigNum (strict)"("Visible"="Gate Width: Time / Percent") -> ()  [unwired: 2 in, 2 out]
                n241 = property on="Target" class="DigNum (strict)"("Visible"="Gate Width: Time / Percent") -> ()  [unwired: 2 in, 2 out]
                n242 = Not(x="Gate Width: Time / Percent") -> (.not. x?=w458:bool)
                n243 = property on="Setpoint" class="DigNum (strict)"("Visible"=w458) -> ()  [unwired: 2 in, 2 out]
                n244 = property on="Current" class="DigNum (strict)"("Visible"=w458) -> ()  [unwired: 2 in, 2 out]
                n245 = property on="Current" class="DigNum (strict)"("Visible"=w458) -> ()  [unwired: 2 in, 2 out]
                n246 = property on="Setpoint" class="DigNum (strict)"("Visible"=w458) -> ()  [unwired: 2 in, 2 out]
              }
              frame #1 {
                # "Frechem: Did not change"
                n247 = local read "Internal / External"() -> (w461:bool)
                n248 = local read "# Triggers vs Freq/Time"() -> (w460:bool)
                n249 = Not(x=w461) -> (.not. x?=w459:bool)
                n250 = property on="Set Count Time" class="Bool"("Visible"=w459) -> ()  [unwired: 2 in, 2 out]
                n251 = Or(x=w459, y=w460) -> (x .or. y?=w465:bool)
                n252 = Not(x=w460) -> (.not. x?=w462:bool)
                n253 = And(x=w461, y=w460) -> (x .and. y?=w464:bool)
                n254 = property on="Setpoint" class="DigNum (strict)"("Visible"=w464) -> ()  [unwired: 2 in, 2 out]
                n255 = property on="Current" class="DigNum (strict)"("Visible"=w464) -> ()  [unwired: 2 in, 2 out]
                n256 = property on="Current" class="DigNum (strict)"("Visible"=w465) -> ()  [unwired: 2 in, 2 out]
                n257 = property on="Setpoint" class="DigNum (strict)"("Visible"=w465) -> ()  [unwired: 2 in, 2 out]
                n258 = And(x=w461, y=w462) -> (x .and. y?=w463:bool)
                n259 = property on="Set Time & Freq." class="Bool"("Visible"=w464) -> ()  [unwired: 2 in, 2 out]
                n260 = property on="Setpoint" class="DigNum (strict)"("Visible"=w463) -> ()  [unwired: 2 in, 2 out]
                n261 = property on="Current" class="DigNum (strict)"("Visible"=w463) -> ()  [unwired: 2 in, 2 out]
                n262 = property on="# Triggers vs Freq/Time" class="Bool (strict)"("Visible"=w461) -> ()  [unwired: 2 in, 2 out]
                n263 = property on="Set # of Triggers" class="Bool"("Visible"=w463) -> ()  [unwired: 2 in, 2 out]
              }
            }
            n264 = local write "Update visible/hidden"(FALSE ("Update visiible/hidden")) -> ()
          }
          event "Set # Periods": Value Change {
            # "This allows you to update the number of periods to be taken while the device is running\nwithout being reinitialized."
            n265 = event-data() -> ()  [unwired: 2 out]
            n266 = call "Set Num Periods.vi"("# of periods"=w466, "Set # Periods"="Set # Periods", "Error In"=w468, "VISA resource name"=w469) -> ("Error Out"=w475:errorcluster, "VISA resource name out"=w474:refnum<visa-resource-name>)  [unwired: 6 in]
            n267 = call "Get Number Periods.vi"("error in (no error)"=w475, "VISA resource name"=w474) -> ("error out"=w470:errorcluster, "# Periods"=→"Current":dbl, "VISA resource name out"=w471:refnum<visa-resource-name>)  [unwired: 7 in]
          }
          event "Set Dwell Time": Value Change {
            # "This allows you to update the dwell time\nwithout reinitialization."
            n268 = event-data() -> ()  [unwired: 7 out]
            n269 = call "Set Dwell Time.vi"("Error In"=w484, "Dwell time"=w482, "Set # Periods"="Set Dwell Time", "VISA resource name"=w485) -> ("Error Out"=w480:errorcluster, "VISA resource name out"=w481:refnum<visa-resource-name>)  [unwired: 6 in]
            n270 = call "Get Dwell Time.vi"("error in (no error)"=w480, "VISA resource name"=w481) -> ("error out"=w477:errorcluster, "output"=→"Current":dbl[unit], "VISA resource name out"=w478:refnum<visa-resource-name>)  [unwired: 7 in]
          }
          event "Read Buffer Data": Value Change {
            # "Read data VI courtesy of Paul Henning on the\nNational Instruments forum."
            n271 = event-data() -> ()  [unwired: 7 out]
            n272 = Add(x=w489, y=w488) -> (x+y=w486:dbl[unit])
            n273 = flat-sequence {
              tunnel: w500 -> [w512]
              tunnel: w502 -> [w511]
              tunnel: w504 -> [w510]
              tunnel: w506 -> [w509]
              tunnel: [w509] -> w499
              tunnel: [w510] -> w498
              tunnel: [w511] -> w497
              tunnel: [w512] -> w496
              tunnel: [w508] -> w491
              tunnel: w490 -> [w508]
              tunnel: [w507] -> w487
              tunnel: w486 -> [w507]
              tunnel: w499 -> [w522]
              tunnel: w498 -> [w520]
              tunnel: w497 -> [w518]
              tunnel: w496 -> [w516]
              tunnel: [w521] -> w495
              tunnel: [w519] -> w494
              tunnel: [w517] -> w493
              tunnel: w491 -> [w514]
              tunnel: w487 -> [w513]
              tunnel: [w565] -> w501
              tunnel: [w562] -> w503
              tunnel: [w563] -> w505
              tunnel: w495 -> [w560]
              tunnel: w494 -> [w564]
              tunnel: w493 -> [w565]
              frame #0 {
              }
              frame #1 {
                n274 = case shown="True" TRUE {
                  tunnel: w522 -> [w523 w534]
                  tunnel: [w523 w533] -> w521
                  tunnel: w520 -> [w524 w532]
                  tunnel: [w524 w531] -> w519
                  tunnel: w518 -> [w525 w530]
                  tunnel: [w525 w529] -> w517
                  tunnel: w516 -> [_ w528]
                  tunnel: w514 -> [_ w527]
                  tunnel: w513 -> [_ w526]
                  frame False {
                  }
                  frame True {
                    n275 = flat-sequence {
                      tunnel: w528 -> [w553]
                      tunnel: w534 -> [w536]
                      tunnel: w532 -> [w551]
                      tunnel: w530 -> [w552]
                      tunnel: w527 -> [w549]
                      tunnel: [w535] -> w533
                      tunnel: [w551] -> w531
                      tunnel: [w552] -> w529
                      tunnel: w526 -> [w547]
                      frame #0 {
                        n276 = Index Array(array=w549, index=0) -> (element=w546:timestamp)
                        n277 = Number To Decimal String(number="GPIB Address") -> (decimal integer string=w557:string)  [unwired: 1 in]
                        n278 = call "Read Data.vi"("Channel Number"=1, "GPIB Address"=w557, "Number of Datapoints"=w553) -> ("Data"=w550:i32[])
                        n279 = call "Read Data.vi"("Channel Number"=0, "GPIB Address"=w557, "Number of Datapoints"=w553) -> ("Data"=w541:i32[])
                        n280 = node(w547) -> (w538:dbl)
                        n281 = Bundle By Name("Y"=w550, "t0"=w546, "dt"=w538) -> (w539:waveform(i32))  [unwired: 1 in]
                        n282 = To Double Precision Float(number=w541) -> (double precision float=w540:dbl[])
                        n283 = Bundle By Name("Y"=w540, "t0"=w546, "dt"=w538) -> (w545:waveform(dbl))  [unwired: 1 in]
                        n284 = Build Array(w545, w539) -> (w544:waveform(dbl)[])
                        n285 = call-poly <vilib>:"Export Waveforms to Spreadsheet File.vi"("header? (write header:T)"=FALSE, "error in (no error)"=w536, "multiple time columns? (single:F)"=FALSE, "waveforms"=w544, "file path (dialog if empty)"="file path") -> ("error out"=w535:errorcluster)  [unwired: 5 in, 1 out]
                      }
                    }
                  }
                }
              }
              frame #2 {
                w558 = dbl[] [] ("History Data")
                n286 = property on="Counter A" class="WFChart (strict)"(error in=w560, "History Data"=w558) -> (error out=w559:errorcluster)  [unwired: 1 in, 1 out]
                n287 = property on="Counter B" class="WFChart (strict)"(error in=w559, "History Data"=w558) -> (error out=w561:errorcluster)  [unwired: 1 in, 1 out]
                n288 = call "Reset Counters.vi"("error in (no error)"=w561, "VISA resource name"=w564) -> ("error out"=w563:errorcluster, "VISA resource name out"=w562:refnum<visa-resource-name>)  [unwired: 8 in]
              }
            }
            n289 = local write "Read Buffer Data"(FALSE ("Read Buffer Data")) -> ()
          }
          event "Start Scan": Value Change {
            # "This allows you to start and stop a scan with the counts being from the buffer for display."
            n290 = event-data() -> ()  [unwired: 7 out]
            n291 = flat-sequence {
              tunnel: w587 -> [w822]
              tunnel: w586 -> [w817]
              tunnel: w585 -> [w818]
              tunnel: [w820] -> w596
              tunnel: [w821] -> w595
              tunnel: [w822] -> w594
              tunnel: [w827] -> w593
              tunnel: [w825] -> w592
              tunnel: [w824] -> w591
              tunnel: w596 -> [w828]
              tunnel: w595 -> [w826]
              tunnel: w594 -> [w824]
              tunnel: [w830] -> w589
              tunnel: w593 -> [w830]
              tunnel: w592 -> [w829]
              tunnel: [w831] -> w588
              tunnel: w591 -> [w831]
              tunnel: [w829] -> w590
              frame #0 {
                n292 = call "Clear Status Byte.vi"("error in (no error)"=w818, "VISA resource name"=w817) -> ("error out"=w819:errorcluster, "VISA resource name out"=w816:refnum<visa-resource-name>)  [unwired: 8 in]
                n293 = call "Reset Counters.vi"("error in (no error)"=w819, "VISA resource name"=w816) -> ("error out"=w820:errorcluster, "VISA resource name out"=w821:refnum<visa-resource-name>)  [unwired: 8 in]
              }
              frame #1 {
                n294 = call "Start button.vi"("error in (no error)"=w828, "VISA resource name"=w826) -> ("error out"=w827:errorcluster, "VISA resource name out"=w825:refnum<visa-resource-name>)  [unwired: 8 in]
                n295 = Get Date/Time In Seconds() -> (seconds since 1Jan1904=→"Scan Start Time":timestamp)
              }
              frame #2 {
                n296 = local write "Start Scan"(FALSE ("Read Channels")) -> ()
              }
            }
            n297 = call <vilib>:"DAQmx Start Task.vi"("task/channels in"=w567) -> ("task out"=w566:refnum<k21>)  [unwired: 13 in, 1 out]
            n298 = call <vilib>:"DAQmx Start Task.vi"("task/channels in"=w569) -> ("task out"=w568:refnum<k21>)  [unwired: 13 in, 1 out]
            n299 = while {
              tunnel: [w636] -> w583
              tunnel: w590 -> [w631]
              tunnel: [w637] -> w582
              tunnel: w589 -> [w632]
              tunnel: [w638] -> w584
              tunnel: w588 -> [w635]
              tunnel: [w633] -> w581
              shift-right: [w629] -> _
              shift-left: 0.0 -> [w623]
              tunnel: w578 -> [w628]
              tunnel: w579 -> [w620]
              shift-right: [w618] -> w576
              shift-left: w577 -> [w617]
              tunnel: w566 -> [w615]
              tunnel: [w613] -> w575
              tunnel: [w611] -> w574
              tunnel: w568 -> [w597]
              tunnel: w573 -> [w609]
              shift-right: [w605] -> _
              shift-left: dbl[] [] ("data") -> [w606]
              shift-right: [w604] -> _
              shift-left: 0.0 -> [w607]
              shift-right: [w599] -> _
              shift-left: 0.0 -> [w600]
              stop <- w624 stop-if-true
              n300 = flat-sequence {
                tunnel: w631 -> [w655]
                tunnel: [w655] -> w642
                tunnel: w632 -> [w654]
                tunnel: [w654] -> w641
                tunnel: w635 -> [w653]
                tunnel: [w653] -> w634
                tunnel: ["Stop Scan"] -> w625
                tunnel: [w651] -> w621
                tunnel: w620 -> [w651]
                tunnel: [w650] -> w616
                tunnel: w615 -> [w650]
                tunnel: [w649] -> w610
                tunnel: w597 -> [w649]
                tunnel: w607 -> [w648]
                tunnel: w606 -> [w645]
                tunnel: [w647] -> w602
                tunnel: [w646] -> w601
                tunnel: w600 -> [w646]
                tunnel: [w677] -> w640
                tunnel: w642 -> [w679]
                tunnel: w641 -> [w678]
                tunnel: [w683] -> w639
                tunnel: w634 -> [w683]
                tunnel: [w676] -> w630
                tunnel: w623 -> [w675]
                tunnel: [w674] -> w622
                tunnel: w621 -> [w672]
                tunnel: [w671] -> w619
                tunnel: w617 -> [w670]
                tunnel: w616 -> [w668]
                tunnel: [w667] -> w614
                tunnel: [w666] -> w612
                tunnel: w610 -> [w664]
                tunnel: w609 -> [w663]
                tunnel: [w662] -> w608
                tunnel: [w661] -> w603
                tunnel: w602 -> [w659]
                tunnel: w601 -> [w657]
                tunnel: [w656] -> w598
                tunnel: [w792] -> w638
                tunnel: [w791] -> w637
                tunnel: w640 -> [w796]
                tunnel: w639 -> [w795]
                tunnel: [w794] -> w636
                tunnel: w624 -> [w797]
                tunnel: [w790] -> w633
                tunnel: w630 -> [w793]
                tunnel: [w789] -> w629
                tunnel: w622 -> [w789]
                tunnel: w619 -> [w788]
                tunnel: [w788] -> w618
                tunnel: w614 -> [w785]
                tunnel: [w785] -> w613
                tunnel: w612 -> [w784]
                tunnel: [w784] -> w611
                tunnel: w608 -> [w783]
                tunnel: [w783] -> w605
                tunnel: [w782] -> w604
                tunnel: w603 -> [w782]
                tunnel: [w781] -> w599
                tunnel: w598 -> [w781]
                frame #0 {
                  n301 = Index Array(array=w645, index=0) -> (element=w643:dbl)
                  n302 = Add(x=w643, y=w648) -> (x+y=w647:dbl)
                }
                frame #1 {
                  n303 = flat-sequence {
                    tunnel: w678 -> [w691]
                    tunnel: w679 -> [w690]
                    tunnel: [w694] -> w682
                    tunnel: [w692] -> w681
                    tunnel: [w689] -> w680
                    tunnel: [w688] -> w673
                    tunnel: w672 -> [w688]
                    tunnel: [w687] -> w669
                    tunnel: w668 -> [w687]
                    tunnel: [w686] -> w665
                    tunnel: w664 -> [w686]
                    tunnel: [w685] -> w660
                    tunnel: w659 -> [w685]
                    tunnel: [w684] -> w658
                    tunnel: w657 -> [w684]
                    tunnel: w682 -> [w713]
                    tunnel: w681 -> [w712]
                    tunnel: w680 -> [w714]
                    tunnel: w675 -> [w709]
                    tunnel: [w711] -> w676
                    tunnel: [w710] -> w677
                    tunnel: [w708] -> w674
                    tunnel: w673 -> [w707]
                    tunnel: [w706] -> w671
                    tunnel: w670 -> [w705]
                    tunnel: w669 -> [w704]
                    tunnel: [w703] -> w667
                    tunnel: [w702] -> w666
                    tunnel: w665 -> [w701]
                    tunnel: w663 -> [w700]
                    tunnel: [w699] -> w662
                    tunnel: [w698] -> w661
                    tunnel: w660 -> [w697]
                    tunnel: w658 -> [w696]
                    tunnel: [w695] -> w656
                    frame #0 {
                      n304 = call "Query Status Byte.vi"("error in (no error)"=w691, "VISA resource name"=w690) -> ("error out"=w692:errorcluster, "Status Register"=w693:T6, "VISA resource name out"=w694:refnum<visa-resource-name>)  [unwired: 7 in]
                      n305 = Unbundle(w693) -> ("Data Ready"=w689:bool)  [unwired: 10 out]
                    }
                    frame #1 {
                      n306 = case shown="True" w714 {
                        tunnel: w713 -> [w728 w749]
                        tunnel: w712 -> [w727 w748]
                        tunnel: [w727 w746] -> w710
                        tunnel: [w728 w747] -> w711
                        tunnel: w709 -> [w726 w743]
                        tunnel: [w726 w742] -> w708
                        tunnel: w707 -> [_ w740]
                        tunnel: [w725 w738] -> w706
                        tunnel: w705 -> [w725 w737]
                        tunnel: w704 -> [w724 w736]
                        tunnel: [w724 w734] -> w703
                        tunnel: [w721 w732] -> w702
                        tunnel: w701 -> [w722 w731]
                        tunnel: w700 -> [w723 _]
                        tunnel: [w719 _] -> w699
                        tunnel: [w718 _] -> w698
                        tunnel: w697 -> [w718 w730]
                        tunnel: w696 -> [w717 w729]
                        tunnel: [w715 _] -> w695
                        frame False {
                          n307 = Add(x=1.0, y=w717) -> (x+y=w715:dbl)
                          n308 = call-poly <vilib>:"DAQmx Read.vi"("task/channels in"=w722, "number of samples per channel"=w723, "timeout"=10.0) -> ("task out"=w721:refnum<k21>, "data"=w719:dbl[])  [unwired: 10 in, 1 out]
                        }
                        frame True {
                          n309 = flat-sequence {
                            tunnel: w749 -> [w768]
                            tunnel: w748 -> [w767]
                            tunnel: [w764] -> w745
                            tunnel: [w762] -> w744
                            tunnel: [w758] -> w741
                            tunnel: w740 -> [w758]
                            tunnel: [w757] -> w739
                            tunnel: w736 -> [w756]
                            tunnel: [w755] -> w735
                            tunnel: [w753] -> w733
                            tunnel: w731 -> [w753]
                            tunnel: w730 -> [w750]
                            tunnel: w729 -> [w751]
                            tunnel: [w779] -> w746
                            tunnel: [w780] -> w747
                            tunnel: w745 -> [w777]
                            tunnel: w744 -> [w778]
                            tunnel: w743 -> [w775]
                            tunnel: [w774] -> w742
                            tunnel: w741 -> [_]
                            tunnel: w739 -> [w773]
                            tunnel: [w772] -> w738
                            tunnel: w737 -> [w771]
                            tunnel: w735 -> [w770]
                            tunnel: [w770] -> w734
                            tunnel: w733 -> [w769]
                            tunnel: [w769] -> w732
                            frame #0 {
                              n310 = call "Query Counts.vi"("error in (no error)"=w767, "Read B?"=FALSE, "VISA resource name"=w768) -> ("error out"=w763:errorcluster, "Counts"=→"Counter A":dbl, "VISA resource name out"=w765:refnum<visa-resource-name>)  [unwired: 6 in]
                              n311 = call-poly <vilib>:"DAQmx Read.vi"("task/channels in"=w756) -> ("task out"=w755:refnum<k21>, "data"=→"Wavemeter":dbl)  [unwired: 12 in, 1 out]
                              n312 = call "Query Counts.vi"("error in (no error)"=w763, "Read B?"=TRUE, "VISA resource name"=w765) -> ("error out"=w762:errorcluster, "Counts"=→"Counter B":dbl, "VISA resource name out"=w764:refnum<visa-resource-name>)  [unwired: 6 in]
                              n313 = Divide(x=w750, y=w751) -> (x/y=→"PMT":dbl)
                              n314 = Get Date/Time In Seconds() -> (seconds since 1Jan1904=w757:timestamp)
                            }
                            frame #1 {
                              n315 = Build Array (concatenate)(w771, w773) -> (w772:timestamp[])
                              n316 = call "Clear Status Byte.vi"("error in (no error)"=w778, "VISA resource name"=w777) -> ("error out"=w779:errorcluster, "VISA resource name out"=w780:refnum<visa-resource-name>)  [unwired: 8 in]
                              n317 = Add(x=w775, y=1.0) -> (x+y=w774:dbl)
                            }
                          }
                        }
                      }
                    }
                  }
                }
                frame #2 {
                  n318 = case shown="True" w797 {
                    tunnel: w796 -> [w804 w813]
                    tunnel: w793 -> [w803 w814]
                    tunnel: w795 -> [w805 w815]
                    tunnel: [w805 w815] -> w794
                    tunnel: [w801 w808] -> w792
                    tunnel: [w802 w809] -> w791
                    tunnel: [w800 w810] -> w790
                    tunnel: [FALSE TRUE] -> w787
                    tunnel: [TRUE FALSE] -> w786
                    frame False {
                      n319 = call "Query Status Byte.vi"("error in (no error)"=w804, "VISA resource name"=w803) -> ("error out"=w801:errorcluster, "Status Register"=w800:T6, "VISA resource name out"=w802:refnum<visa-resource-name>)  [unwired: 7 in]
                    }
                    frame True {
                      n320 = call "Stop button.vi"("error in (no error)"=w813, "VISA resource name"=w814) -> ("error out"=w811:errorcluster, "VISA resource name out"=w812:refnum<visa-resource-name>)  [unwired: 8 in]
                      n321 = call "Query Status Byte.vi"("error in (no error)"=w811, "VISA resource name"=w812) -> ("error out"=w808:errorcluster, "Status Register"=w810:T6, "VISA resource name out"=w809:refnum<visa-resource-name>)  [unwired: 7 in]
                    }
                  }
                  "Scan Finished" <- w787
                  "Scanning" <- w786
                }
              }
              n322 = To Double Precision Float(number=w628) -> (double precision float=w627:dbl)
              n323 = Equal?(x=w623, y=w627) -> (x = y?=w626:bool)
              n324 = Or(x=w625, y=w626) -> (x .or. y?=w624:bool)
              "Current Period" <- w623
            }
          }
        }
        n325 = call <vilib>:"Simple Error Handler.vi"("error in (no error)"=w55) -> ("error out"=w54:errorcluster)  [unwired: 1 in, 7 out]
      }
      n326 = call <vilib>:"DAQmx Clear Task.vi"("task in"=w23) -> ()  [unwired: 14 in, 1 out]
      n327 = call <vilib>:"DAQmx Clear Task.vi"("task in"=w24) -> ()  [unwired: 14 in, 1 out]
    }
    frame #2 {
    }
  }
  "error out" <- w5
